vi "Master Control Loops.vi"() -> ()   [LabVIEW 2009]
uses:
  lib/Control Loop/Control Loop State.ctl
  lib/Data Access Objects/Control Loop/PID Controls.ctl
  lib/MixedMode/Mixed Mode States.ctl
  lib/MixedMode/Mixed Mode Convergence Status.ctl
  lib/MixedMode/Stiffness Matrix.ctl
  lib/Control Loop/Measurements.ctl
  lib/Data Access Objects/Metadata/LBCB Position.ctl
  lib/Control Loop/Limit Settings.ctl
  lib/Control Loop/Limit Matrix.ctl
  lib/Limits/Within Limits Matrix.ctl
  lib/Limits/Actuator Faults.ctl
  lib/Limits/Cart Disp Faults.ctl
  lib/Limits/Cart Force Faults.ctl
  lib/MixedMode/Target Data.ctl
  lib/MixedMode/Mixed Mode Cartesian Data.ctl
  lib/Autobalance/Autobalance Status Data.ctl
  lib/Apps/Yes No Button.ctl
  lib/Autobalance/Autobalance Stage.ctl
  lib/Autobalance/Autobalance Data Point.ctl
  lib/Data Access Objects/Mixed Mode/Force Control Parameters.ctl
  lib/Control Loop/Mixed Mode Hold Data type.ctl
  lib/Control Loop/Act & Cart Commands.ctl
  lib/Data Access Objects/Autobalance/Autobalance Control Parameters.ctl
  lib/Data Access Objects/Metadata/Cartesian Point.ctl
  lib/Global Data/Jacobian Stiffness Column.ctl
  lib/Global Data/Jacobian Stiffness Column Id.ctl
  lib/Control Loop/MM Result Actions.ctl
  lib/Data Access Objects/Metadata/DAO Actions.ctl
  lib/Apps/App Status Actions.ctl
  lib/Control Loop/Parameters Changes.ctl
  lib/Control Loop/Parameter Change States.ctl
  lib/Data Access Objects/Metadata/LBCB Number.ctl
  lib/MixedMode/Messages/Mixed Mode Command.ctl
  lib/MixedMode/Mixed Mode Command Action.ctl
  lib/MixedMode/Ramp Time Tuple.ctl
  lib/MixedMode/Messages/Mixed Mode Status.ctl
  lib/Autobalance/Autobalance State.ctl
  lib/Data Access Objects/Metadata/Persistant DAO Actions.ctl
  lib/Data Access Objects/Application/Number Of LBCBs.ctl
  lib/Global Data/Transactions/Dataset Transaction Id.ctl
  lib/Global Data/Transactions/Dataset Source.ctl
  lib/Global Data/Transactions/Dataset Type.ctl
  lib/Logging/Command or Stiffness Updates.ctl
  lib/Global Data/Command Or Stiffness Update Type.ctl
  lib/Data Access Objects/Global Cache/Global Cache.vi
  lib/Logging/LogFileType.ctl
  lib/DAQ IO/Daq Actions.ctl
  lib/Launcher/NoPanelAppTypes.ctl
  lib/Launcher/Launcher Actions.ctl
panel:
  out "MM Result Actions":T1
  out "Commands":T2[](array[typedef])
  out "Stiffness Jacobian Column":T3[](array[typedef])
  out "Target":T5[](array[typedef])
  out "Cart Individual Cmds":dbl[][](array[numeric])=[[0.015224103858920254, 0.016374115079328375, 0.0001743188568230551, 0.03971045114557009, 0.007082336209989981, 0.009859079687370698, 8.685887933911959, 1.9897804119684945, 4.857688782335148, 93.30834661628205, -5.911514458784602, -1.446477360303783]]
  out "Cart Meas. Disp & Forces":dbl[][](array[numeric])=[[0.015224103858920254, 0.016374115079328375, 0.0001743188568230551, 0.03971045114557009, 0.007082336209989981, 0.009859079687370698, 8.685887933911959, 1.9897804119684945, 4.857688782335148, 93.30834661628205, -5.911514458784602, -1.446477360303783]]
  out "Force Groups":T6[](array[typedef])
  in  "AB Parameters":T7={"Number of Samples"=0, "Delay After Cmd"=0, "Maximum Command"=0.0, "1/4 Linear Range"=0.5}
  out "Increment Limits":T2[](array[typedef])
  out "Hold Data":T8[](array[typedef])
  in  "L2 Ctrl Loop In Actuator":dbl[](array[numeric])
  out "Rigid Connection":bool
  out "Force Parameters":T9
  out "Stiffness Limits":dbl[][][](array[numeric])
  out "L2 Autobalance Out":T10[](array[typedef])
  out "L2 Cmd  Volts":dbl[](array[numeric])
  out "L2 Ctrl Loop Out Actuator":dbl[](array[numeric])=[0.012801822908652838, 0.012801822908652838, 7.98290599846041e-06, 8.154359441903125e-06, 8.154359441903125e-06, 8.154359441903125e-06]
  in  "Monitor Loop Time":u32
  in  "Volts LVDT & LC":dbl[][](array[numeric])
  out "L1 Autobalance Out":T10[](array[typedef])
  out "Collecting DAQ Samples":bool
  out "DAQ Volts":dbl[](array[numeric])=[-5.059315779335383, -5.016629198362524, -5.097891313865665, -5.092890991738198, -5.1138932889519, -4.974194835814303, 0.24442110332308561, 0.2508540081873783, -0.00045656932832031883, -0.0010919008583725697, -0.001119467422792373, -0.001138029771633142, 0.051584220664617125, 0.05637080163747566, -0.0007913138656640637, 0.023009008261802286, -0.021593288951899364, 0.0027051641856972383, -5.059665406563526, -5.018353952939143, -5.097893414204858, -5.0928919356893525, -5.11389113151188, -4.974191443340161, 0.24267296718237016, 0.2422302353042843, -0.0004670710242903981, -0.0011032282722249686, -0.0010935781425555466, -0.0010973200819313358, 0.05123459343647403, 0.05464604706085686, -0.0007934142048580796, 0.02300806431064792, -0.02159113151187963, 0.0027085566598390553, 0.048884220664617124, 0.04853459343647403, 0.050170801637475664, 0.04844604706085686, -9.131386566406377e-05, -9.341420485807962e-05]
  in  "Volt Logger Time":u32
  out "All Stopped":bool
  out "Previous Target":T14[](array[typedef])
  out "Iterative Target":T5[](array[typedef])
  out "Mixed Mode":i32
  out "Status Changes":i32
  out "L2 Control Rate":i32
  out "DAQ Started":bool
  out "Current Target":T5[](array[typedef])
  out "Logging Directory":path
  out "Auto Balance Error Tolerance":dbl[][](array[numeric])=[[0.01, 0.01, 0.01, 0.01, 0.01, 0.01]]
  in  "Hold Period":bool
  in  "Averaging":bool
  out "L1 Ctrl Loop State":T15
  out "Max Increment":dbl[][](array[numeric])
  out "Jacobian Gain":dbl[][](array[numeric])
  out "Force Error Range":dbl[][](array[numeric])
  out "L2 I Gain":dbl[](array[numeric])=[0.3, 0.3, 0.3, 0.3, 0.3, 0.3]
  in  "L2 PID On":bool
  in  "Limits Check":T16[](array[typedef])
  out "L2 P Gain":dbl[](array[numeric])
  out "L2 I Const":dbl[](array[numeric])
  in  "Ramp Time":u32
  out "Limits":T20[](array[typedef])
  out "Position":T22[](array[typedef])
  out "Measurements":T23[](array[typedef])
  out "Stiffness Jacobian":cluster{T24}[](array[cluster])
  out "Convergence Status":T25[](array[typedef])
  out "MixedModeStates":T26
  out "PID Control":T27[](array[typedef])
  in  "L1 PID On":bool
  out "L1 P Gain":dbl[](array[numeric])
  out "L1 I Gain":dbl[](array[numeric])=[0.3, 0.3, 0.3, 0.3, 0.3, 0.3]
  out "L1 I Const":dbl[](array[numeric])
  out "LBCB 1 Control Loop Force Limit":bool
  out "L2 Ctrl Loop State":T15
  out "L1 Cmd  Volts":dbl[](array[numeric])
  out "L1 Ctrl Loop Out Actuator":dbl[](array[numeric])=[0.012801822908652838, 0.012801822908652838, 7.98290599846041e-06, 8.154359441903125e-06, 8.154359441903125e-06, 8.154359441903125e-06]
  out "L1 Control Rate":i32=50 caption="Control Rate"
  in  "L1 Ctrl Loop In Actuator":dbl[](array[numeric])
  out "Number of \nExternal \nChannels":i32
  out "DAQ Enabled":bool
  in  "App Running":bool
  out "DAQ Rate":i32=2 caption="Control Rate"
  out "Servo Error":dbl[][](array[numeric])=[[-0.014471871278962644, -0.0027477897622864888, 0.03594582291831433, -0.006177356244415369, -0.000527948512754489, 0.04718526152757189]]
  out "Actuator Meas. Disp & Forces":dbl[][](array[numeric])=[[0.015224103858920254, 0.016374115079328375, 0.0001743188568230551, 0.03971045114557009, 0.007082336209989981, 0.009859079687370698, 8.685887933911959, 1.9897804119684945, 4.857688782335148, 93.30834661628205, -5.911514458784602, -1.446477360303783]]
  out "External Sensors":dbl[](array[numeric])
  out "DAQ Overflow":bool
  # "(Volts)"
  # "Cmd"
  # "Servo"
  # "Cmd"
  # "Servo"
  # "Cmd"
  # "Servo"
  # "Cmd"
  # "Servo"
  # "(inch)"
  # "X"
  # "(inch)"
  # "Y"
  # "(inch)"
  # "Z"
  # "Xglobal = T*Xlocal"
  # "Continuous"
  # "Hold"
types:
  T1 = typedef "MM Result Actions.ctl" = enum16{"Nop", "Set Command", "Check Limits", "Send Command", "Store Prev Reading", "Averaging On", "Averaging Off", "Hold On", "Hold Off", "PID Hold On", "PID Hold Off", "Clear Increment Faults", "Set Initial Position"}
  T2 = typedef "Act & Cart Commands.ctl" = cluster{"Act Cmd":dbl[], "Cart Cmd":dbl[]}
  T3 = typedef "Jacobian Stiffness Column.ctl" = cluster{"Id":T4, "Column":dbl[]}
  T4 = typedef "Jacobian Stiffness Column Id.ctl" = enum16{"dDx", "dDy", "dDz", "dRx", "dRy", "dRz"}
  T5 = typedef "Target Data.ctl" = cluster{"Displacements":dbl[], "Command Type":enum16{"<None>", "Displacement", "Force"}[], "Forces":dbl[]}
  T6 = typedef "Cartesian Point.ctl" = cluster{"Dx":dbl, "Dy":dbl, "Dz":dbl, "Rx":dbl, "Ry":dbl, "Rz":dbl}
  T7 = typedef "Autobalance Control Parameters.ctl" = cluster{"Number of Samples":i32, "Delay After Cmd":i32, "Maximum Command":dbl, "1/4 Linear Range":dbl}
  T8 = typedef "Mixed Mode Hold Data type.ctl" = cluster{"Displacements":dbl[], "Forces":dbl[], "Displacement \nCommands":dbl[]}
  T9 = typedef "Force Control Parameters.ctl" = cluster{"Use Force Error Range Ratios":bool, "Use Group Priorities":bool, "Multi Command Update":bool, "Steps per Stiffness \nMeasurement":i32}
  T10 = typedef "Autobalance Status Data.ctl" = cluster{"IsBalanced":T11, "Autobalance Stage":T12, "High":T13, "Low":T13, "Balanced \nCmd":dbl}
  T11 = typedef "Yes No Button.ctl" = bool
  T12 = typedef "Autobalance Stage.ctl" = enum16{"Coarse", "Fine", "Backing Up", "Done"}
  T13 = typedef "Autobalance Data Point.ctl" = cluster{"cCmd":dbl, "cServo":dbl, "pCmd":dbl, "pServo":dbl}
  T14 = typedef "Mixed Mode Cartesian Data.ctl" = cluster{"Displacements":dbl[], "Forces":dbl[]}
  T15 = typedef "Control Loop State.ctl" = enum16{"Idle", "Off", "Reset Autobalancing", "Autobalancing", "Set Command", "Ready for Control", "On"}
  T16 = typedef "Within Limits Matrix.ctl" = cluster{"Act Disp":T17, "Act Force":T17, "Act Incr":T17, "Cart Disp":T18, "Cart Force":T19, "Cart Incr":T18}
  T17 = typedef "Actuator Faults.ctl" = cluster{"X1":bool, "X2":bool, "Y1":bool, "Z1":bool, "Z2":bool, "Z3":bool}
  T18 = typedef "Cart Disp Faults.ctl" = cluster{"Dx":bool, "Dy":bool, "Dz":bool, "Rx":bool, "Ry":bool, "Rz":bool}
  T19 = typedef "Cart Force Faults.ctl" = cluster{"Fx":bool, "Fy":bool, "Fz":bool, "Mx":bool, "My":bool, "Mz":bool}
  T20 = typedef "Limit Settings.ctl" = cluster{"Actuator Force Limits":T21, "Actuator Stroke Limits":T21, "Cartesian Disp Limit":T21, "Cartesian Force Limit":T21, "Command Voltage Limit":T21}
  T21 = typedef "Limit Matrix.ctl" = dbl[][]
  T22 = typedef "LBCB Position.ctl" = cluster{"Motion Center":dbl[], "Transformation Matrix":dbl[][]}
  T23 = typedef "Measurements.ctl" = cluster{"Act Disp":dbl[], "Act Forces":dbl[], "Cart Disp":dbl[], "Cart Forces":dbl[]}
  T24 = typedef "Stiffness Matrix.ctl" = dbl[][]
  T25 = typedef "Mixed Mode Convergence Status.ctl" = cluster{"IsConverged":bool[], "Force Errors":dbl[], "Controlling DOF":bool[]}
  T26 = typedef "Mixed Mode States.ctl" = enum16{"Init", "Wait For DAQ", "Idle", "Start Initial Position", "Initial Position", "Start Initial Ramp", "Run Initial Ramp", "Start Iterative Stage", "Convergence Check", "Update Stiffness Jacobian", "Update Command", "Start Iterative Ramp", "Run Iterative Ramp", "Start Iterative Stabilize", "Iterative Stabilize", "Start Iterative Holding", "Iterative Holding", "Start Stabilize", "Stabilize", "Start Hold", "Holding", "Done", "Aborting", "Exit", "Nop"}
  T27 = typedef "PID Controls.ctl" = cluster{"I-Control":bool, "Ctrl Mode":bool}
  T28 = typedef "Command Or Stiffness Update Type.ctl" = cluster{"Target":T5[], "Stiffness":T3[], "Command || Stiffness Update":T29}
  T29 = typedef "Command or Stiffness Updates.ctl" = enum16{"Command Update", "Iterative Command Update", "Stiffness Update"}
  T30 = typedef "Dataset Transaction Id.ctl" = cluster{"Dataset Source":T31, "Dataset Type":T32, "Hold":T11, "Volts":T11, "Tag":string}
  T31 = typedef "Dataset Source.ctl" = enum16{"LBCB 1", "LBCB 2", "Combined", "External Sensors"}
  T32 = typedef "Dataset Type.ctl" = enum16{"LVDT", "Load Cell", "Actuator Command", "Servo Error", "Displacement Command", "Displacement", "Force"}
  T33 = typedef "Number Of LBCBs.ctl" = enum16{"1", "2"}
  T34 = cluster{"Act Disp":dbl[], "Act Forces":dbl[], "Cart Disp":dbl[], "Cart Forces":dbl[]}
  T35 = typedef "LBCB Number.ctl" = enum16{"LBCB1", "LBCB2"}
  T36 = typedef "Persistant DAO Actions.ctl" = enum16{"Init", "Get", "Set", "Load", "Save"}
  T37 = typedef "Autobalance State.ctl" = enum16{"Init", "Send High ", "Wait High", "Read High Start", "Read High", "Send Low", "Wait Low", "Read Low Start", "Read Low", "Publish", "Calculate", "Done"}
  T38 = typedef "Ramp Time Tuple.ctl" = cluster{"Ramp":dbl, "Stab":dbl, "Hold":dbl}
  T39 = typedef "Mixed Mode Command Action.ctl" = enum16{"Start Command", "Stop", "Exit", "No Op", "Start Acquisition", "Measure Initial Position"}
  T40 = typedef "Mixed Mode Status.ctl" = cluster{"LBCB Target":T5[], "MixedModeStates":T26, "LBCB Convergence":T25[], "LBCB Measurements":T14[]}
  T41 = typedef "Mixed Mode Command.ctl" = cluster{"Command":T39, "Ramp Times":cluster{"Initial":T38, "Iterative":T38}, "LBCB1":T5, "LBCB2":T5}
  T42 = typedef "Parameters Changes.ctl" = cluster{"Change State":T43, "LBCB Number":T35}
  T43 = typedef "Parameter Change States.ctl" = enum16{"Mixed Mode", "Control Loop", "Limits", "Application", "Stiffness Jacobian", "Start DAQ", "Reset Auto-Balance", "Set Command", "Enable Control", "Disable Control", "Position", "Stop Application"}
  T44 = typedef "DAO Actions.ctl" = enum16{"Init", "Get", "Set"}
  T45 = typedef "Actuator Matrix.ctl" = cluster{"Lower":T46, "Upper":T46}
  T46 = typedef "Actuator Point.ctl" = cluster{"X1":dbl, "X2":dbl, "Y1":dbl, "Z1":dbl, "Z2":dbl, "Z3":dbl}
  T47 = typedef "Cartesian Matrix.ctl" = cluster{"Lower":T6, "Upper":T6}
  T48 = typedef "App Parameters.ctl" = cluster{"Monitor Loop":T49, "Ramp Time":T49, "Log Loop":T49, "TCP to DAQ":T49, "Logging Directory":path, "Log File Size (MBytes)":i64, "Volt Logging Loop":T49, "2 LBCB Archiving Mode":bool}
  T49 = typedef "Timing Parameters.ctl" = cluster{"Interval":dbl, "Rate ":dbl}
  T50 = typedef "LBCB Settings.ctl" = cluster{"Size":T51, "Type":T52}
  T51 = typedef "LBCB Size.ctl" = enum16{"1/5th-scale LBCB", "Full-scale LBCB", "Portable LBCB"}
  T52 = typedef "LBCB Type.ctl" = enum16{"X Actuators On The Left", "X Actuators On The Right"}
  T53 = typedef "Cartesian Force Vector.ctl" = cluster{"Fx":dbl, "Fy":dbl, "Fz":dbl, "Mx":dbl, "My":dbl, "Mz":dbl}
  T54 = typedef "Calibration Settings.ctl" = cluster{"Command Sensitivity":dbl[], "Servo Error Offset":dbl[], "LVDT Sensitivity":dbl[], "LVDT Offset":dbl[], "Load Cell Offsets":dbl[], "Load Cell Sensitivity":dbl[]}
  T55 = typedef "App Status Actions.ctl" = enum16{"Init", "Get Status", "Running", "Control", "Autobalanced", "Data Acquisition", "Set App State", "DAQ Started", "Set LBCB State", "Set All", "Set Cont Logging", "Set Step Logging", "Set MM Logging", "Set Volt Logging", "Set DAQ Link"}
  T56 = typedef "Ramp Time Input.ctl" = cluster{"Directional":T57, "Iterative":T57}
  T57 = typedef "Ramp Control.ctl" = cluster{"Ramp":dbl, "Stabilize":dbl, "Hold":dbl}
  T58 = typedef "App Status.ctl" = cluster{"Running":bool, "Controlling L2":bool, "Autobalance L2":bool, "Data Acquisition":bool, " App State":T59, "DAQ Started":bool, "LBCB 1 State":T60, "LBCB 2 State":T60, "Controlling L1":bool, "Autobalance L1":bool, "Continuous Logging":bool, "Step Logging":bool, "Voltage Logging":bool, "Mixed Mode Logging":bool, "DAQ Link":bool}
  T59 = typedef "AppStates.ctl" = enum16{"Starting OM", "Initializing Displays", "Setting up Archiving", "Setting Up DAQ Channels", "Start DAQ", "DAQ Starting", "Controlling LBCBs", "Stopping OM"}
  T60 = typedef "Lbcb Control Loop States.ctl" = enum16{"Idle", "Start Selected", "Load Last Command", "Start Autobalancing", "Autobalancing", "Control Loop Initialized", "Control Enabled"}
  T61 = cluster{"Act Disp":dbl[], "Act Forces":dbl[], "Cart Disp":dbl[], "Cart Forces":dbl[]}[]
  T62 = typedef "Daq Actions.ctl" = enum16{"Init", "Send Commands", "Get Responses", "Stop"}
  T63 = enum16{"open", "replace", "create", "open or create", "replace or create", "replace or create with confirmation"}
  T64 = typedef "LogFileType.ctl" = enum16{"Continuous", "Step", "Volts", "Offsets", "DLL  Errors", "Snapshot", "Commands", "StiffnessUpdates", "End List"}
  T65 = typedef "NoPanelAppTypes.ctl" = enum16{"NTCP Socket", "Data Archiving", "DAQ Link", "Control Loops", "Cmd Disp Diffs", "LBCB Data", "Limits", "Mixed Mode Widget", "Offsets"}
  T66 = typedef "Launcher Actions.ctl" = enum16{"Launch", "Stop All", "Stop", "Kill", "Running?", "Init"}
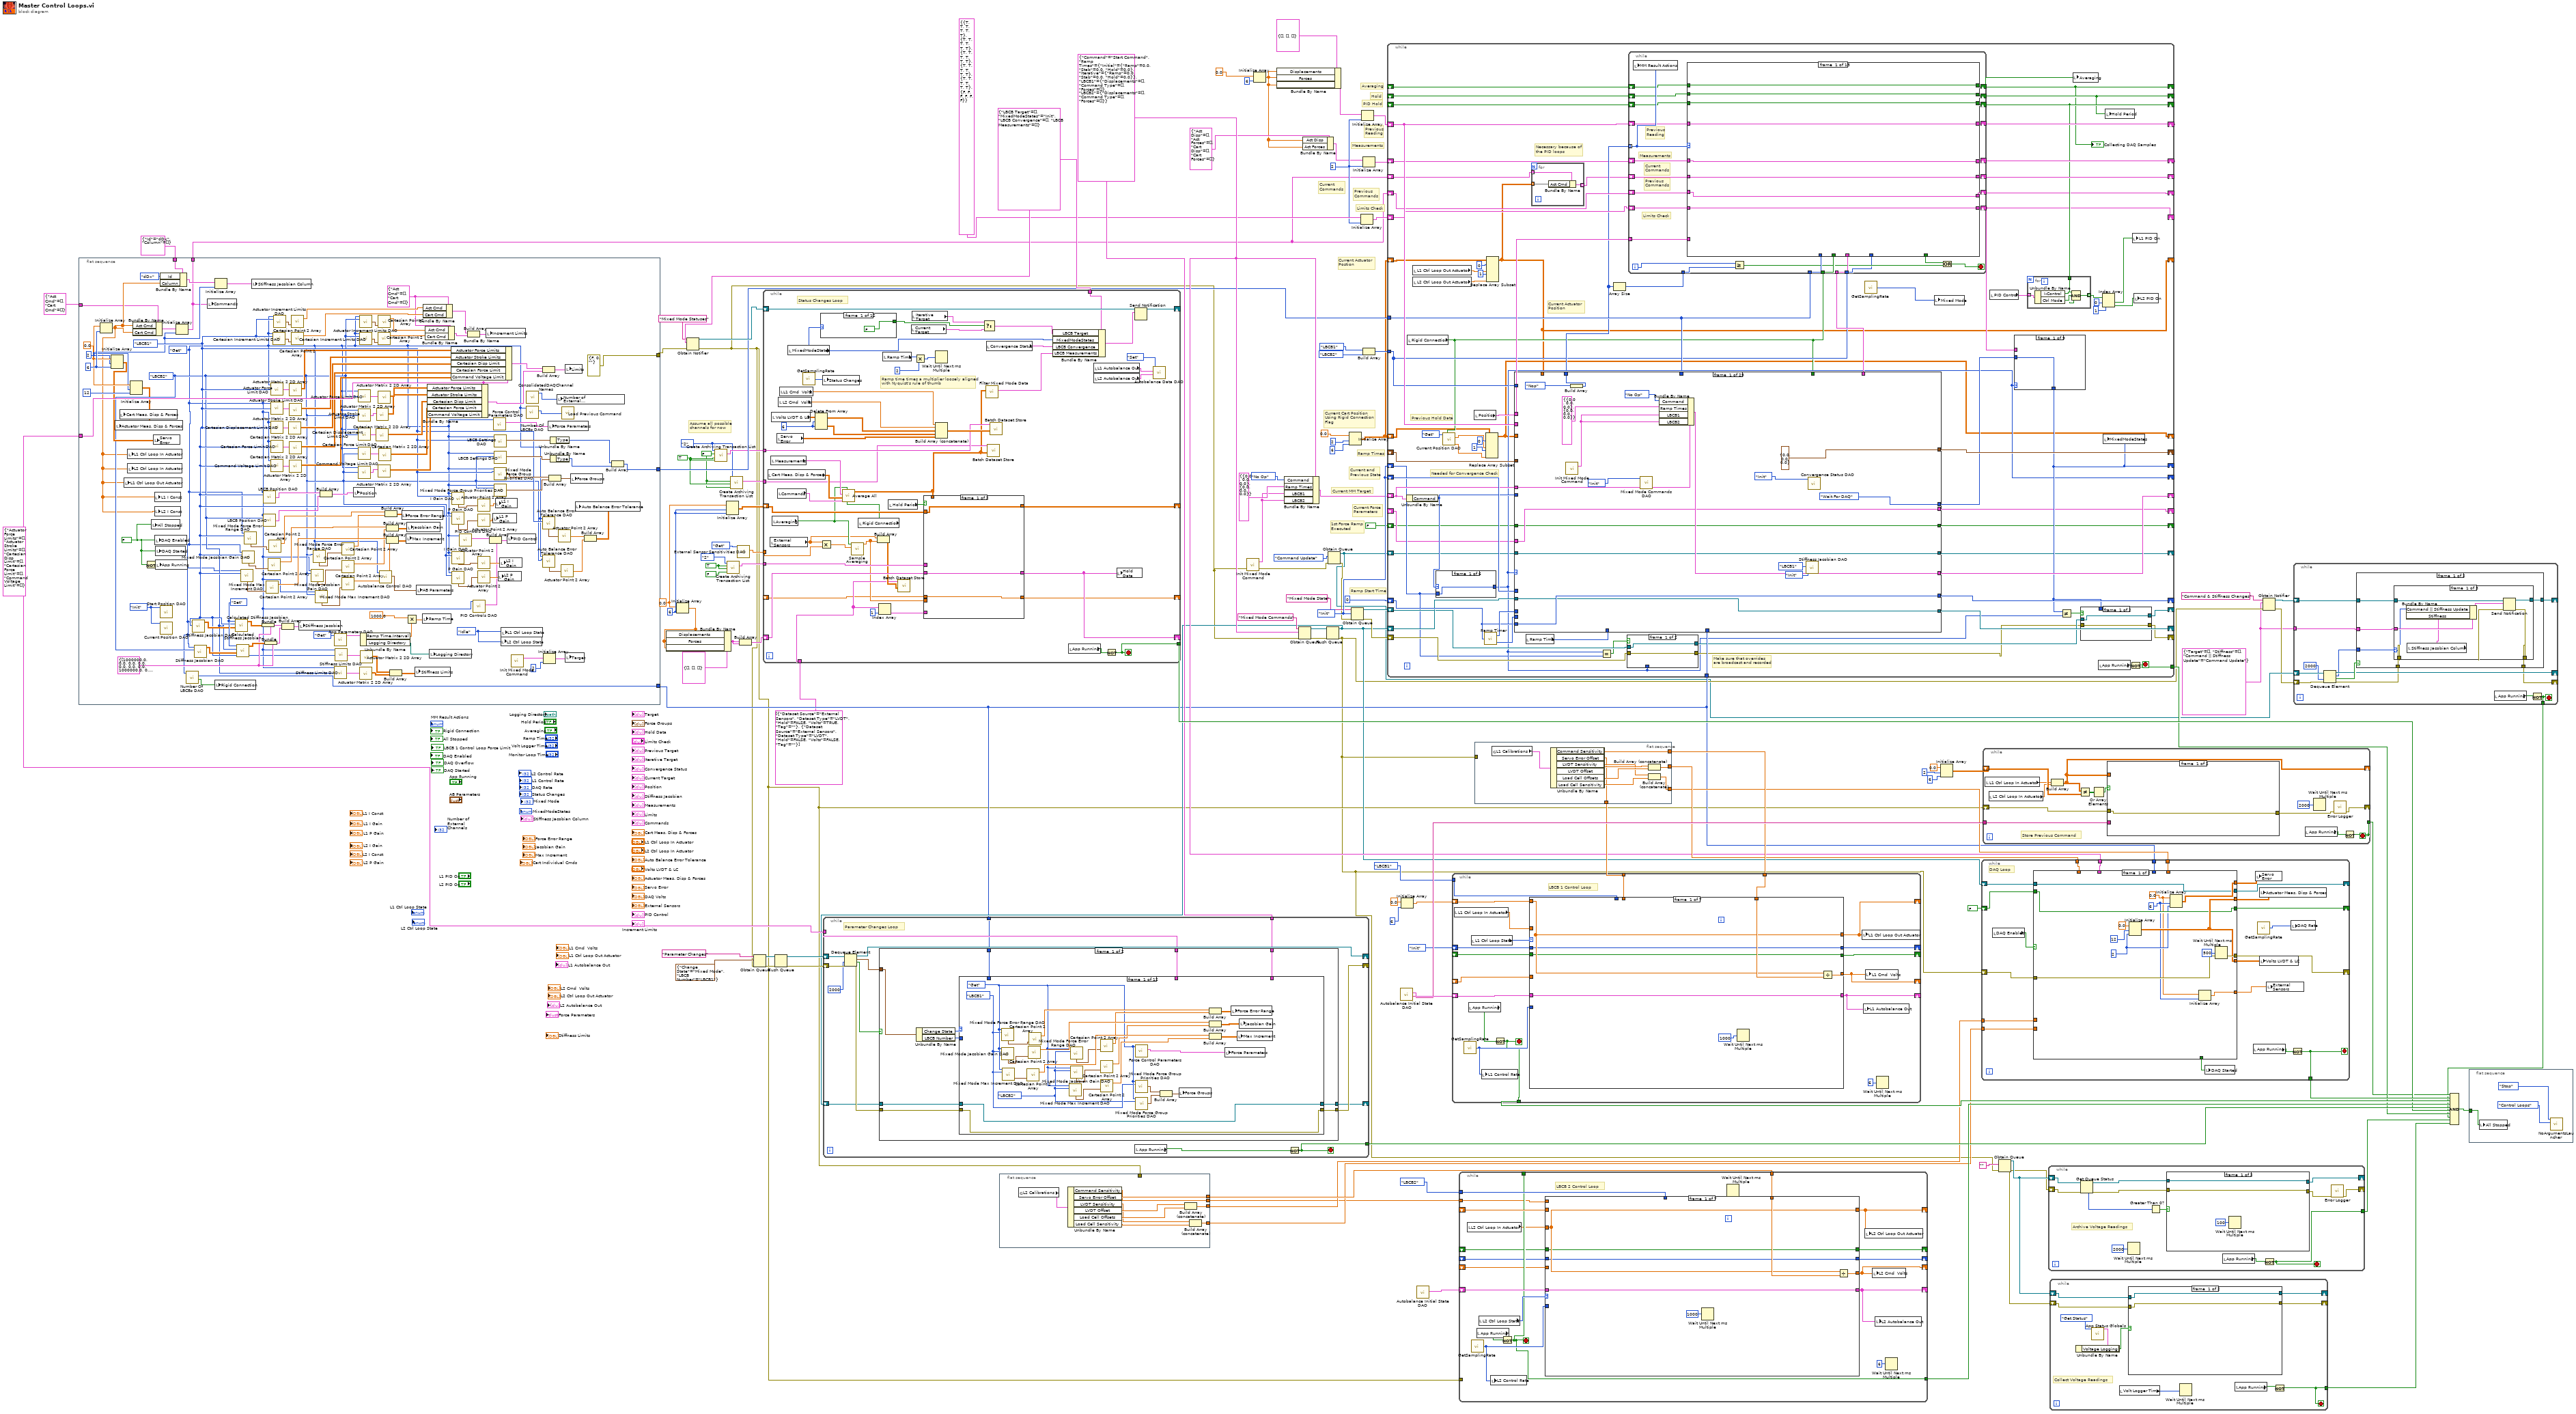
[diagram p0: block diagram]
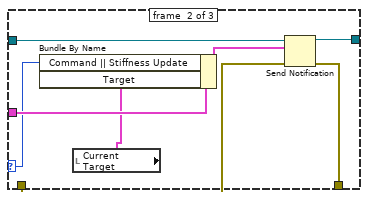
[diagram p2: hidden frame]
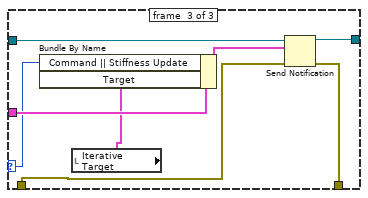
[diagram p3: hidden frame]
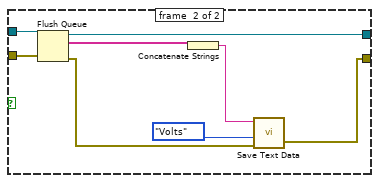
[diagram p5: hidden frame]
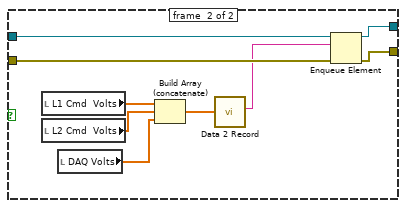
[diagram p6: hidden frame]
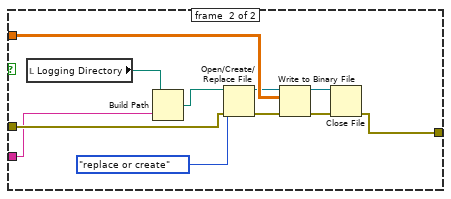
[diagram p7: hidden frame]
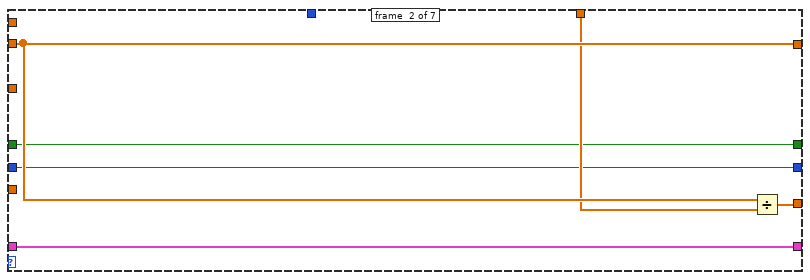
[diagram p8: hidden frame]
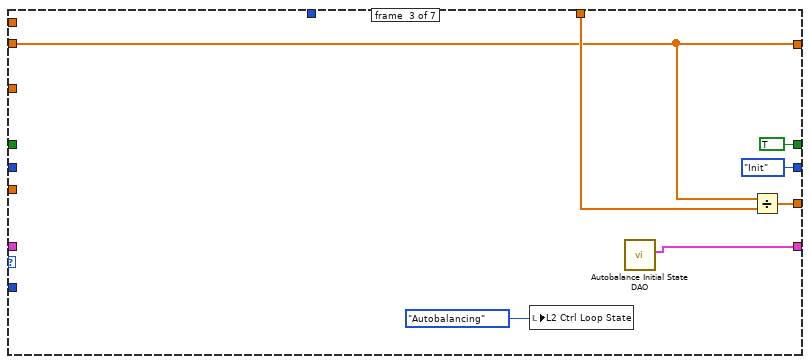
[diagram p9: hidden frame]
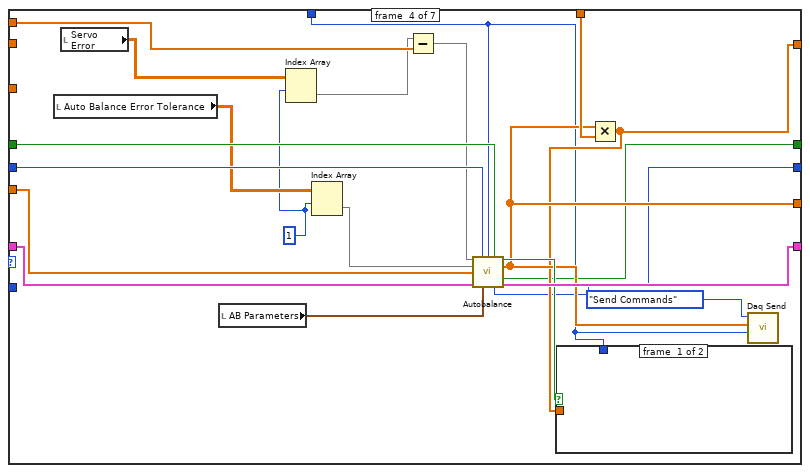
[diagram p10: hidden frame]
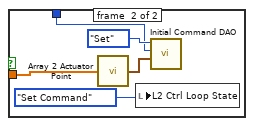
[diagram p11: hidden frame]
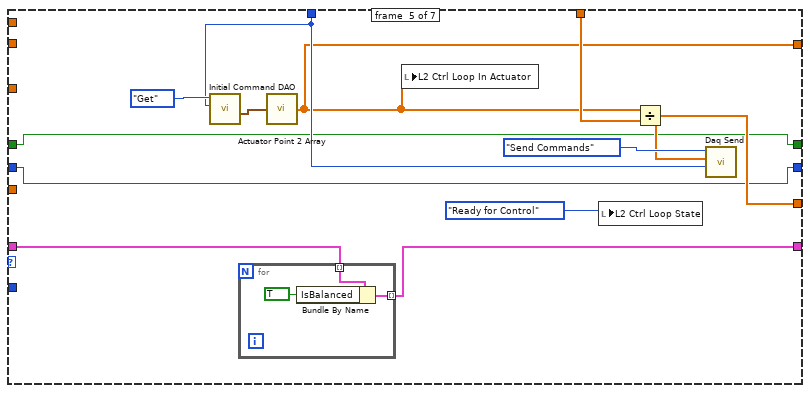
[diagram p12: hidden frame]
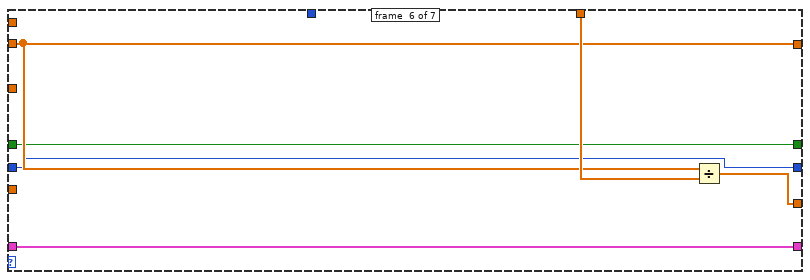
[diagram p13: hidden frame]
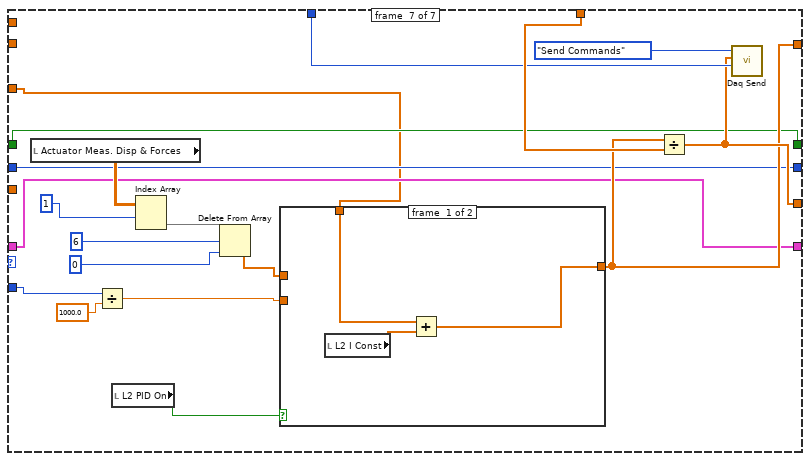
[diagram p14: hidden frame]
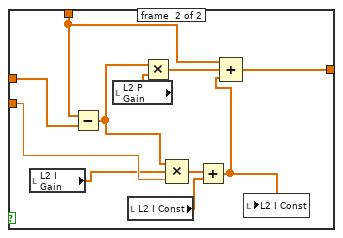
[diagram p15: hidden frame]
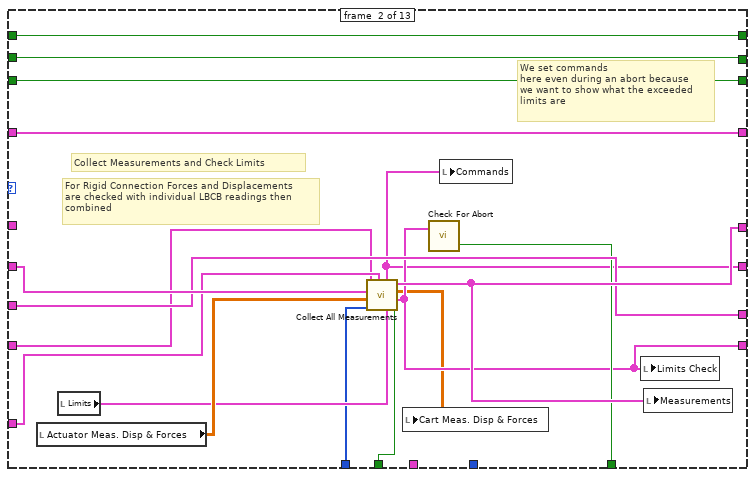
[diagram p16: hidden frame]
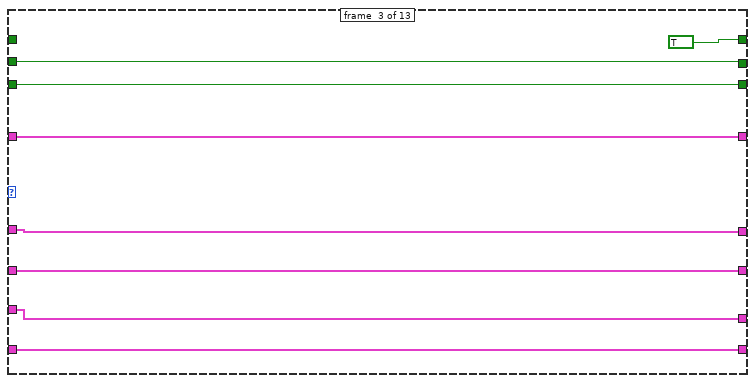
[diagram p17: hidden frame]
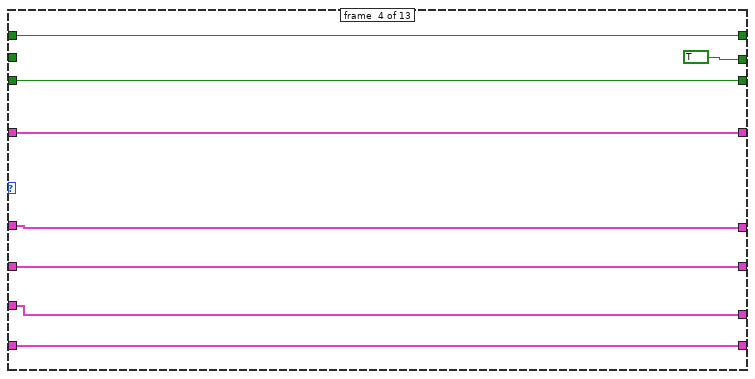
[diagram p18: hidden frame]
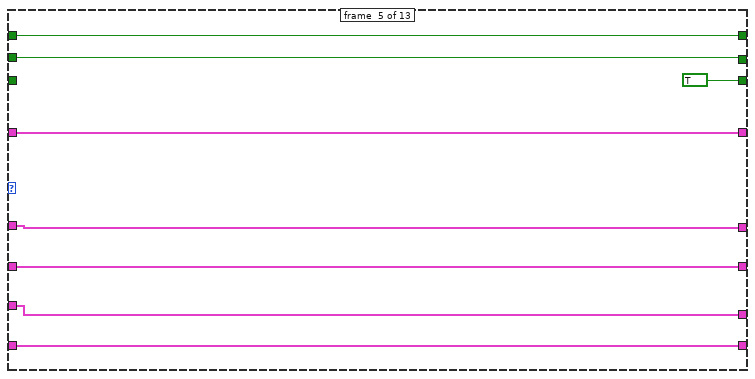
[diagram p19: hidden frame]
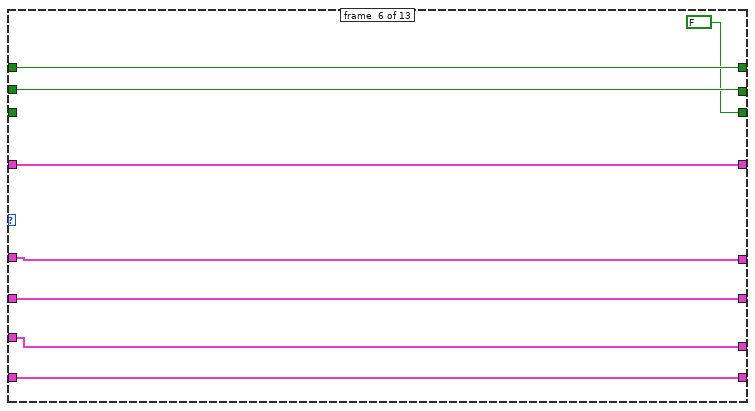
[diagram p20: hidden frame]
diagram:
  w3 = T28 {"Target"=[], "Stiffness"=[], "Command || Stiffness Update"=enum."Command Update"} ("Command || Stiffness Update")
  w20 = TRUE ("Combined LBCBs")
  w17 = Number_Of_LBCBs."2" ("Number of LBCBs")
  w13 = T11 TRUE ("Hold")
  w18 = T11 FALSE ("Hold")
  w23 = 0.0 ("element")
  w24 = 6 ("dimension size")
  w44 = 2 ("dimension size")
  w66 = T20 {"Actuator Force Limits"=[], "Actuator Stroke Limits"=[], "Cartesian Disp Limit"=[], "Cartesian Force Limit"=[], "Command Voltage Limit"=[]} ("L1  Limits")
  w104 = T40 {"LBCB Target"=[], "MixedModeStates"=enum."Init", "LBCB Convergence"=[], "LBCB Measurements"=[]} ("Mixed Mode Status")
  w64 = T41 {"Command"=enum."Start Command", "Ramp Times"={"Initial"={"Ramp"=0.0, "Stab"=0.0, "Hold"=0.0}, "Iterative"={"Ramp"=0.0, "Stab"=0.0, "Hold"=0.0}}, "LBCB1"={"Displacements"=[], "Command Type"=[], "Forces"=[]}, "LBCB2"={"Displacements"=[], "Command Type"=[], "Forces"=[]}} ("Mixed Mode Command")
  w111 = Mixed_Mode_States."Init" ("MixedModeStates")
  # "Assume all possible\nchannels for now"
  # "Current Actuator\nPostion"
  # "Current Cart Position\nUsing Rigid Connection\nFlag"
  # "1st Force Ramp\nExecuted"
  # "Current Force\nParameters"
  # "Previous\nCommands"
  # "Limits Check"
  # "Ramp Start Time"
  # "PID Hold"
  # "Hold"
  # "Averaging"
  # "Previous\nReading"
  # "Current \nCommands"
  # "Measurements"
  # "Current MM Target"
  # "Current and\nPrevious State"
  # "Ramp Times"
  n1 = flat-sequence {
    tunnel: [errorcluster {"status"=FALSE, "code"=0, "source"=""} ("error out")] -> w69
    tunnel: w66 -> [w207]
    tunnel: [w156] -> w46
    tunnel: [w151] -> w45
    tunnel: [w116] -> w43
    tunnel: T3 {"Id"=enum."dDx", "Column"=[]} ("Jacobian Stiffness Column") -> [w125]
    tunnel: T2 {"Act Cmd"=[], "Cart Cmd"=[]} ("Data") -> [w120]
    frame #0 {
      w127 = DAO_Actions."Init" ("DAO Actions")
      w129 = T2 {"Act Cmd"=[], "Cart Cmd"=[]} ("Data")
      w173 = cluster{T24} {[[1000000.0, 0.0, 0.0, 0.0, 0.0, 0.0], [0.0, 1000000.0, 0.0, 0.0, 0.0, 0.0], [0.0, 0.0, 1000000.0, 0.0, 0.0, 0.0], [0.0, 0.0, 0.0, 1000000.0, 0.0, 0.0], [0.0, 0.0, 0.0, 0.0, 1000000.0, 0.0], [0.0, 0.0, 0.0, 0.0, 0.0, 1000000.0]]} ("Cluster")
      w126 = 2 ("dimension size")
      w210 = Control_Loop_State."Idle" ("L1 Ctrl Loop State")
      w177 = 6 ("dimension size")
      w176 = 0.0 ("element")
      w137 = LBCB_Number."LBCB2" ("ID")
      w138 = LBCB_Number."LBCB1" ("ID")
      w136 = Persistant_DAO_Actions."Get" ("Actuator Force Limit Actions")
      w214 = FALSE
      w230 = Persistant_DAO_Actions."Set" ("Actions")
      n2 = Initialize Array(w176, w177) -> (w123:dbl[])
      n3 = Initialize Array(w176, w126, w177) -> (w141:dbl[][])
      n4 = local write "L1 Ctrl Loop Out Actuator"(w123) -> ()
      n5 = local write "L1 Ctrl Loop In Actuator"(w123) -> ()
      n6 = local write "L2 Ctrl Loop In Actuator"(w123) -> ()
      n7 = Initialize Array(w176, w126, 12 ("dimension size")) -> (w128:dbl[][])
      n8 = local write "Actuator Meas. Disp & Forces"(w128) -> ()
      n9 = local write "Cart Meas. Disp & Forces"(w128) -> ()
      n10 = Bundle By Name(cluster=w120, "Act Cmd"=w123, "Cart Cmd"=w123) -> (w150:T2)
      n11 = Not(x=w214) -> (.not. x?=w228:bool)
      n12 = local write "All Stopped"(w214) -> ()
      n13 = local write "Servo Error"(w141) -> ()
      n14 = local write "L1 I Const"(w123) -> ()
      n15 = local write "L2 I Const"(w123) -> ()
      n16 = local write "DAQ Enabled"(w214) -> ()
      n17 = local write "DAQ Started"(w214) -> ()
      n18 = local write "App Running"(w228) -> ()
      n19 = call "Start Position DAO.vi"("DAO Actions"=w127) -> ()  [unwired: 9 in, 2 out]
      n20 = call "Current Position DAO.vi"("Actions"=w127) -> ()  [unwired: 9 in, 2 out]
      n21 = Bundle By Name(cluster=w125, "Id"=Jacobian_Stiffness_Column_Id."dDx", "Column"=w123) -> (w122:T3)
      n22 = Initialize Array(w150, w126) -> (w116:T2[])
      n23 = call "Number Of LBCBs DAO.vi"("Actions"=w136) -> ("Rigid Connection Out"=w157:bool, "Number of\nLBCBs Out"=w156:T33)  [unwired: 4 in, 5 out]
      n24 = call "Stiffness Jacobian DAO.vi"("LBCB Number"=w138, "Actions"=w136) -> ("Stiffness Jacobian Out"=w229:T24)  [unwired: 3 in, 6 out]
      n25 = call "Stiffness Jacobian DAO.vi"("LBCB Number"=w137, "Actions"=w136) -> ("Stiffness Jacobian Out"=w231:T24)  [unwired: 3 in, 6 out]
      n26 = local write "Commands"(w116) -> ()
      n27 = local write "Rigid Connection"(w157) -> ()
      n28 = Initialize Array(w122, w126) -> (w121:T3[])
      n29 = call "Calculated Stiffness Jacobian.vi"("Stiffness Jacobian In"=w229, "LBCB Number"=w138, "Actions"=w230) -> ("Stiffness Jacobian Out"=w175:T24)  [unwired: 1 in, 7 out]
      n30 = call "Calculated Stiffness Jacobian.vi"("Stiffness Jacobian In"=w231, "LBCB Number"=w137, "Actions"=w230) -> ("Stiffness Jacobian Out"=w174:T24)  [unwired: 1 in, 7 out]
      n31 = call "Mixed Mode Max Increment DAO.vi"("Max Increment Actions"=w136, "LBCB Number"=w138) -> ("Max Increment Out"=w238:T6)  [unwired: 3 in, 10 out]
      n32 = call "Mixed Mode Jacobian Gain DAO.vi"("Jacobian Gain Actions"=w136, "LBCB Number"=w138) -> ("Jacobian Gain Out"=w237:T6)  [unwired: 3 in, 10 out]
      n33 = call "Mixed Mode Force Error Range DAO.vi"("Force Error Range Actions"=w136, "LBCB Number"=w138) -> ("Force Error Range Out"=w236:T6)  [unwired: 3 in, 10 out]
      n34 = local write "Stiffness Jacobian Column"(w121) -> ()
      n35 = Bundle(cluster=w173, w175) -> (w172:cluster{T24})
      n36 = call "LBCB Position DAO.vi"("LBCB Settings Actions"=w136, "LBCB Number"=w138) -> ("LBCB Position Output"=w235:T22)  [unwired: 3 in, 10 out]
      n37 = call "LBCB Position DAO.vi"("LBCB Settings Actions"=w136, "LBCB Number"=w137) -> ("LBCB Position Output"=w185:T22)  [unwired: 3 in, 10 out]
      n38 = Bundle(cluster=w173, w174) -> (w171:cluster{T24})
      n39 = call "Cartesian Point 2 Array.vi"("Cart Disp"=w238) -> ("Array"=w232:dbl[])  [unwired: 2 out]
      n40 = call "Cartesian Point 2 Array.vi"("Cart Disp"=w237) -> ("Array"=w233:dbl[])  [unwired: 2 out]
      n41 = call "Cartesian Point 2 Array.vi"("Cart Disp"=w236) -> ("Array"=w234:dbl[])  [unwired: 2 out]
      n42 = call "Actuator Force Limit DAO.vi"("Actuator Force Limit Actions"=w136, "ID"=w138) -> ("Actuator Force Limits Out"=w206:T45)  [unwired: 3 in, 10 out]
      n43 = call "Actuator Stroke Limit DAO.vi"("Actuator Stroke Limit Actions"=w136, "ID"=w138) -> ("Actuator Stroke Limits Out"=w205:T45)  [unwired: 3 in, 10 out]
      n44 = call "Cartesian Displacement Limit DAO.vi"("Cartesian Displacement Limit Actions"=w136, "ID"=w138) -> ("Cartesian Displacement Out"=w200:T47)  [unwired: 3 in, 10 out]
      n45 = call "Cartesian Force Limit DAO.vi"("Cartesian Force Limit Actions"=w136, "ID"=w138) -> ("Cartesian Force Limit Out"=w199:T47)  [unwired: 3 in, 10 out]
      n46 = call "Command Voltage Limit DAO.vi"("Actuator Stroke Limit Actions"=w136, "ID"=w138) -> ("Command Voltage Limit Out"=w204:T45)  [unwired: 3 in, 10 out]
      n47 = call "Cartesian Increment Limits DAO.vi"("Actions"=w136, "LBCB Number"=w138) -> ("Inc Limits Out"=w149:T6)  [unwired: 11 in, 2 out]
      n48 = call "Actuator Increment Limits DAO.vi"("Actions"=w136, "LBCB Number"=w138) -> ("Inc Limits Out"=w140:T46)  [unwired: 11 in, 2 out]
      n49 = Build Array(w172, w171) -> (w170:cluster{T24}[])
      n50 = call "Cartesian Matrix 2 2D Array.vi"("Matrix In"=w200) -> ("Matrix Out"=w188:T21)  [unwired: 10 out]
      n51 = call "Actuator Matrix 2 2D Array.vi"("Matrix In"=w206) -> ("Matrix Out"=w203:T21)  [unwired: 10 out]
      n52 = call "Actuator Matrix 2 2D Array.vi"("Matrix In"=w205) -> ("Matrix Out"=w202:T21)  [unwired: 10 out]
      n53 = call "Cartesian Matrix 2 2D Array.vi"("Matrix In"=w199) -> ("Matrix Out"=w187:T21)  [unwired: 10 out]
      n54 = call "Actuator Matrix 2 2D Array.vi"("Matrix In"=w204) -> ("Matrix Out"=w201:T21)  [unwired: 10 out]
      n55 = call "Cartesian Point 2 Array.vi"("Cart Disp"=w149) -> ("Array"=w133:dbl[])  [unwired: 2 in]
      n56 = call "Cartesian Point 2 Array.vi"("Cart Disp"=w140) -> ("Array"=w135:dbl[])  [unwired: 2 in]
      n57 = local write "Stiffness Jacobian"(w170) -> ()
      n58 = call "Mixed Mode Jacobian Gain DAO.vi"("Jacobian Gain Actions"=w136, "LBCB Number"=w137) -> ("Jacobian Gain Out"=w212:T6)  [unwired: 3 in, 10 out]
      n59 = call "Mixed Mode Force Error Range DAO.vi"("Force Error Range Actions"=w136, "LBCB Number"=w137) -> ("Force Error Range Out"=w211:T6)  [unwired: 3 in, 10 out]
      n60 = call "Mixed Mode Max Increment DAO.vi"("Max Increment Actions"=w136, "LBCB Number"=w137) -> ("Max Increment Out"=w213:T6)  [unwired: 3 in, 10 out]
      n61 = Build Array(w235, w185) -> (w186:T22[])
      n62 = call "App Parameters DAO.vi"("Actions"=Persistant_DAO_Actions."Get") -> ("Application Timing and Logging Out"=w242:T48)  [unwired: 3 in, 7 out]
      n63 = call "Stiffness Limits DAO.vi"("Cartesian Force Limit Actions"=w136, "ID"=w137) -> ("Stiffness Limit Out"=w160:T47)  [unwired: 11 in, 2 out]
      n64 = call "Stiffness Limits DAO.vi"("Cartesian Force Limit Actions"=w136, "ID"=w138) -> ("Stiffness Limit Out"=w162:T47)  [unwired: 11 in, 2 out]
      n65 = call "Cartesian Point 2 Array.vi"("Cart Disp"=w211) -> ("Array"=w183:dbl[])  [unwired: 1 in, 1 out]
      n66 = call "Cartesian Point 2 Array.vi"("Cart Disp"=w212) -> ("Array"=w181:dbl[])  [unwired: 1 in, 1 out]
      n67 = call "Cartesian Point 2 Array.vi"("Cart Disp"=w213) -> ("Array"=w179:dbl[])  [unwired: 1 in, 1 out]
      n68 = local write "Position"(w186) -> ()
      n69 = call "Actuator Force Limit DAO.vi"("Actuator Force Limit Actions"=w136, "ID"=w137) -> ("Actuator Force Limits Out"=w198:T45)  [unwired: 3 in, 10 out]
      n70 = call "Actuator Stroke Limit DAO.vi"("Actuator Stroke Limit Actions"=w136, "ID"=w137) -> ("Actuator Stroke Limits Out"=w197:T45)  [unwired: 3 in, 10 out]
      n71 = call "Cartesian Displacement Limit DAO.vi"("Cartesian Displacement Limit Actions"=w136, "ID"=w137) -> ("Cartesian Displacement Out"=w196:T47)  [unwired: 3 in, 10 out]
      n72 = call "Cartesian Force Limit DAO.vi"("Cartesian Force Limit Actions"=w136, "ID"=w137) -> ("Cartesian Force Limit Out"=w195:T47)  [unwired: 3 in, 10 out]
      n73 = call "Command Voltage Limit DAO.vi"("Actuator Stroke Limit Actions"=w136, "ID"=w137) -> ("Command Voltage Limit Out"=w194:T45)  [unwired: 3 in, 10 out]
      n74 = call "Cartesian Increment Limits DAO.vi"("Actions"=w136, "LBCB Number"=w137) -> ("Inc Limits Out"=w148:T6)  [unwired: 11 in, 2 out]
      n75 = call "Actuator Increment Limits DAO.vi"("Actions"=w136, "LBCB Number"=w137) -> ("Inc Limits Out"=w139:T46)  [unwired: 11 in, 2 out]
      n76 = call "Actuator Matrix 2 2D Array.vi"("Matrix In"=w160) -> ("Matrix Out"=w159:T21)  [unwired: 10 out]
      n77 = Unbundle By Name(w242) -> ("Ramp Time.Interval"=w243:dbl, "Logging Directory"=w239:path)
      n78 = call "Actuator Matrix 2 2D Array.vi"("Matrix In"=w162) -> ("Matrix Out"=w161:T21)  [unwired: 10 out]
      n79 = call "Cartesian Matrix 2 2D Array.vi"("Matrix In"=w196) -> ("Matrix Out"=w191:T21)  [unwired: 10 out]
      n80 = call "Actuator Matrix 2 2D Array.vi"("Matrix In"=w197) -> ("Matrix Out"=w192:T21)  [unwired: 10 out]
      n81 = call "Cartesian Point 2 Array.vi"("Cart Disp"=w148) -> ("Array"=w132:dbl[])  [unwired: 2 in]
      n82 = call "Cartesian Point 2 Array.vi"("Cart Disp"=w139) -> ("Array"=w134:dbl[])  [unwired: 2 in]
      n83 = call "Actuator Matrix 2 2D Array.vi"("Matrix In"=w198) -> ("Matrix Out"=w193:T21)  [unwired: 10 out]
      n84 = call "Actuator Matrix 2 2D Array.vi"("Matrix In"=w194) -> ("Matrix Out"=w189:T21)  [unwired: 10 out]
      n85 = call "Cartesian Matrix 2 2D Array.vi"("Matrix In"=w195) -> ("Matrix Out"=w190:T21)  [unwired: 10 out]
      n86 = call "Autobalance Control DAO.vi"("Persistent DAO Actions"=w136) -> ("Autobalance Control Out"=w146:T7)  [unwired: 8 in, 2 out]
      n87 = Build Array(w234, w183) -> (w184:dbl[][])
      n88 = Build Array(w233, w181) -> (w182:dbl[][])
      n89 = Build Array(w232, w179) -> (w180:dbl[][])
      n90 = Build Array(w161, w159) -> (w158:dbl[][][])
      n91 = local write "Force Error Range"(w184) -> ()
      n92 = local write "Max Increment"(w180) -> ()
      n93 = Multiply(x=1000.0, y=w243) -> (x*y=w240:dbl)
      n94 = local write "Jacobian Gain"(w182) -> ()
      n95 = local write "Stiffness Limits"(w158) -> ()
      n96 = local write "AB Parameters"(w146) -> ()
      n97 = local write "Ramp Time"(w240) -> ()
      n98 = Bundle By Name(cluster=w129, "Act Cmd"=w135, "Cart Cmd"=w133) -> (w131:T2)
      n99 = Bundle By Name(cluster=w129, "Act Cmd"=w134, "Cart Cmd"=w132) -> (w130:T2)
      n100 = Bundle By Name(cluster=w207, "Actuator Force Limits"=w193, "Actuator Stroke Limits"=w192, "Cartesian Disp Limit"=w191, "Cartesian Force Limit"=w190, "Command Voltage Limit"=w189) -> (w166:T20)
      n101 = local write "Logging Directory"(w239) -> ()
      n102 = Bundle By Name(cluster=w207, "Actuator Force Limits"=w203, "Actuator Stroke Limits"=w202, "Cartesian Disp Limit"=w188, "Cartesian Force Limit"=w187, "Command Voltage Limit"=w201) -> (w208:T20)
      n103 = call "I Gain DAO.vi"("I Gain Actions"=w136, "LBCB Number"=w138) -> ("I Gain"=w224:T46)  [unwired: 3 in, 10 out]
      n104 = call "P Gain DAO.vi"("P Gain Actions"=w136, "LBCB Number"=w138) -> ("P Gain"=w225:T46)  [unwired: 3 in, 10 out]
      n105 = call "I Gain DAO.vi"("I Gain Actions"=w136, "LBCB Number"=w137) -> ("I Gain"=w227:T46)  [unwired: 3 in, 10 out]
      n106 = call "P Gain DAO.vi"("P Gain Actions"=w136, "LBCB Number"=w137) -> ("P Gain"=w226:T46)  [unwired: 3 in, 10 out]
      n107 = call "PID Controls DAO.vi"("Actions"=w136) -> ("PID Control  Out"=w165:T27)  [unwired: 3 in, 7 out]
      n108 = Build Array(w131, w130) -> (w147:T2[])
      n109 = call "PID Controls DAO.vi"("Actions"=w136) -> ("PID Control  Out"=w163:T27)  [unwired: 3 in, 7 out]
      n110 = call "Actuator Point 2 Array.vi"("Actuator Point"=w224) -> ("Array"=w223:dbl[])
      n111 = call "Actuator Point 2 Array.vi"("Actuator Point"=w225) -> ("Array"=w222:dbl[])
      n112 = call "Actuator Point 2 Array.vi"("Actuator Point"=w227) -> ("Array"=w221:dbl[])
      n113 = call "Actuator Point 2 Array.vi"("Actuator Point"=w226) -> ("Array"=w220:dbl[])
      n114 = local write "Increment Limits"(w147) -> ()
      n115 = Build Array(w165, w163) -> (w164:T27[])
      n116 = local write "L1 P Gain"(w222) -> ()
      n117 = call "Force Control Parameters DAO.vi"("DAO Actions"=w136) -> ("Force Control Parameters Out"=w142:T9)  [unwired: 8 in, 2 out]
      n118 = call "LBCB Settings DAO.vi"("LBCB Number"=w138, "Actions"=w136) -> ("LBCB Setting Out"=w154:T50)  [unwired: 3 in, 6 out]
      n119 = call "LBCB Settings DAO.vi"("LBCB Number"=w137, "Actions"=w136) -> ("LBCB Setting Out"=w155:T50)  [unwired: 3 in, 6 out]
      n120 = call "Mixed Mode Force Group Priorities DAO.vi"("Force Error Range Actions"=w136, "LBCB Number"=w138) -> ("Force Group Priorities Out"=w145:T53)  [unwired: 11 in, 2 out]
      n121 = call "Mixed Mode Force Group Priorities DAO.vi"("Force Error Range Actions"=w136, "LBCB Number"=w137) -> ("Force Group Priorities Out"=w144:T53)  [unwired: 11 in, 2 out]
      n122 = local write "L1 I Gain"(w223) -> ()
      n123 = local write "L2 P Gain"(w220) -> ()
      n124 = local write "L2 I Gain"(w221) -> ()
      n125 = local write "L2 Ctrl Loop State"(w210) -> ()
      n126 = local write "L1 Ctrl Loop State"(w210) -> ()
      n127 = local write "PID Control"(w164) -> ()
      n128 = call "Init Mixed Mode Command.vi"() -> ("Command Data"=w119:T5)  [unwired: 2 in, 1 out]
      n129 = call "Number Of LBCBs DAO.vi"("Actions"=w136) -> ("Number of\nLBCBs Out"=w209:T33)  [unwired: 4 in, 6 out]
      n130 = call "ConsolidatedDAQChannelNames.vi"() -> ("Number of \nExternal \nChannels 1"=w219:i32)  [unwired: 5 out]
      n131 = call "Auto Balance Error Tolerance DAO.vi"("Auto Balance Increment Actions"=w136, "LBCB Number"=w138) -> ("Auto Balance Error Out"=w217:T46)  [unwired: 3 in, 10 out]
      n132 = Build Array(w208, w166) -> (w167:T20[])
      n133 = call "Auto Balance Error Tolerance DAO.vi"("Auto Balance Increment Actions"=w136, "LBCB Number"=w137) -> ("Auto Balance Error Out"=w218:T46)  [unwired: 3 in, 10 out]
      n134 = Initialize Array(w119, 2 ("dimension size")) -> (w118:T5[])
      n135 = local write "Force Parameters"(w142) -> ()
      n136 = Build Array(w145, w144) -> (w143:T53[])
      n137 = Unbundle By Name(w154) -> ("Type"=w153:T52)
      n138 = Unbundle By Name(w155) -> ("Type"=w152:T52)
      n139 = local write "Number of \nExternal \nChannels"(w219) -> ()
      n140 = call "Actuator Point 2 Array.vi"("Actuator Point"=w217) -> ("Array"=w216:dbl[])
      n141 = call "Actuator Point 2 Array.vi"("Actuator Point"=w218) -> ("Array"=w168:dbl[])
      n142 = call "Load Previous Command.vi"("Number of LBCBs"=w209) -> ()  [unwired: 3 out]
      n143 = local write "Limits"(w167) -> ()
      n144 = local write "Target"(w118) -> ()
      n145 = local write "Force Groups"(w143) -> ()
      n146 = Build Array(w216, w168) -> (w169:dbl[][])
      n147 = local write "Auto Balance Error Tolerance"(w169) -> ()
      n148 = Build Array(w153, w152) -> (w151:T52[])
    }
  }
  n149 = Initialize Array(w23, w24) -> (w41:dbl[])
  n150 = Bundle By Name(cluster=T8 {"Displacements"=[], "Forces"=[], "Displacement \nCommands"=[]} ("element"), "Displacements"=w41, "Forces"=w41, "Displacement \nCommands"=w41) -> (w40:T8)
  n151 = Obtain Notifier(name (unnamed)="Mixed Mode Statuses", notification data type=w104, error in (no error)=w69) -> (notifier out=w105:refnum<notifier>, error out=w9:errorcluster)  [unwired: 1 in, 1 out]
  n152 = call "Create Archiving Transaction List.vi"("Volts Only"=w20, "Combined LBCBs"=w20, "Hold"=w18, "Number of LBCBs"=w17) -> ("Transactions"=w21:T30[])  [unwired: 7 in]
  n153 = Initialize Array(w23, w24, w24) -> (w22:dbl[][])
  n154 = call "Create Archiving Transaction List.vi"("Volts Only"=FALSE, "Combined LBCBs"=w13, "Hold"=w13, "Number of LBCBs"=Number_Of_LBCBs."2") -> ("Transactions"=w16:T30[])  [unwired: 7 in]
  n155 = call "Create Archiving Transaction List.vi"("Volts Only"=w18, "Combined LBCBs"=w20, "Hold"=w18, "Number of LBCBs"=w17) -> ("Transactions"=w19:T30[])  [unwired: 7 in]
  n156 = call "External Sensor Sensitivities DAO.vi"("Persistent DAO Actions"=Persistant_DAO_Actions."Get") -> ("Sensitivities Out"=w70:dbl[])  [unwired: 3 in, 7 out]
  n157 = Build Array(w40, w40) -> (w25:T8[])
  n158 = Obtain Queue(name (unnamed)="Parameter Changes", element data type=T42 {"Change State"=enum."Mixed Mode", "LBCB Number"=enum."LBCB1"} ("Parameter Changes"), error in (no error)=w9) -> (queue out=w113:refnum<queue>, error out=w91:errorcluster)  [unwired: 2 in, 1 out]
  n159 = while {
    shift-right: [w264] -> _
    shift-left: w25 -> [w263]
    tunnel: w70 -> [w294]
    shift-right: [w289] -> _
    shift-left: w105 -> [w290]
    tunnel: w104 -> [w288]
    tunnel: [w284] -> w96
    tunnel: w21 -> [w255]
    tunnel: w16 -> [w266]
    shift-right: [w265] -> _
    shift-left: w22 -> [w262]
    tunnel: T30[] [{"Dataset Source"=enum."External Sensors", "Dataset Type"=enum."LVDT", "Hold"=FALSE, "Volts"=TRUE, "Tag"=""}, {"Dataset Source"=enum."External Sensors", "Dataset Type"=enum."LVDT", "Hold"=FALSE, "Volts"=FALSE, "Tag"=""}] ("Transactions") -> [w253]
    shift-right: [w249] -> _
    shift-left: _ -> [w248]
    tunnel: w19 -> [w247]
    stop <- w284 stop-if-true
    w272 = 6 ("length")
    # "Ramp time times a multiplier loosely aligned\nwith Nyquist's rule of thumb"
    # "Status Changes Loop"
    n160 = local read "Cart Meas. Disp & Forces"() -> (w268:dbl[][])
    n161 = local read "External Sensors"() -> (w257:dbl[])
    n162 = local read "Measurements"() -> (w275:T23[])
    n163 = local read "Volts LVDT & LC"() -> (w273:dbl[][])
    n164 = local read "Averaging"() -> (w258:bool)
    n165 = local read "Servo Error"() -> (w269:dbl[][])
    n166 = local read "Commands"() -> (w260:T2[])
    n167 = local read "L2 Cmd  Volts"() -> (w274:dbl[])
    n168 = local read "L1 Cmd  Volts"() -> (w295:dbl[])
    n169 = local read "MixedModeStates"() -> (w280:T26)
    n170 = call "GetSamplingRate.vi"() -> ("Sampling"=w285:i32)
    n171 = Delete From Array(array=w273, length=w272, index (col)=w272) -> (deleted portion=w270:dbl[][], array with subset deleted=w271:dbl[][])  [unwired: 1 in]
    n172 = Multiply(x=w257, y=w294) -> (x*y=w259:dbl[])
    n173 = case shown="\"Update Command\"" w280 {
      tunnel: [FALSE TRUE TRUE TRUE TRUE TRUE TRUE TRUE TRUE TRUE TRUE TRUE] -> w276
      frame #0 {
      }
      frame #1 {
      }
      frame #2 {
      }
      frame #3 {
      }
      frame #4 {
      }
      frame #5 {
      }
      frame #6 {
      }
      frame #7 {
      }
      frame #8 {
      }
      frame #9 {
      }
      frame #10 {
      }
      frame #11 {
      }
    }
    n174 = local write "Status Changes"(w285) -> ()
    n175 = call "Sample Averaging.vi"("Sample In"=w259, "Averaging"=w258) -> ("Sample Out"=w250:dbl[])  [unwired: 9 in]
    n176 = local read "Rigid Connection"() -> (w245:bool)
    n177 = call "Average All.vi"("Rigid Connection"=w245, "Averaging"=w258, "Commands"=w260, "Individual Measurements"=w268, "Measurements"=w275) -> ("Data"=w246:dbl[][])  [unwired: 6 in]
    n178 = Build Array(w257, w250) -> (w254:dbl[][])
    n179 = Index Array(array=w253, index=1) -> (element=w251:T30)
    n180 = local read "Ramp Time"() -> (w293:u32)
    n181 = local read "Hold Period"() -> (w267:bool)
    n182 = call "Batch Dataset Store.vi"("Data"=w254, "Transactions"=w253) -> ()  [unwired: 9 in, 1 out]
    n183 = local read "Current Target"() -> (w279:T5[])
    n184 = local read "Iterative Target"() -> (w277:T5[])
    n185 = Multiply(x=w293, y=u32 2) -> (x*y=w291:u32)
    n186 = case shown="True" w267 {
      tunnel: w266 -> [_ w304]
      tunnel: [w298 w305] -> w265
      tunnel: w246 -> [_ w307]
      tunnel: [w299 w306] -> w264
      tunnel: w263 -> [w299 _]
      tunnel: w262 -> [w298 _]
      tunnel: w251 -> [_ w303]
      tunnel: w250 -> [_ w302]
      tunnel: [w297 w300] -> w249
      tunnel: w248 -> [w297 _]
      frame #0 {
      }
      frame #1 {
        n187 = call "Filter Hold Data.vi"("Data"=w307) -> ("Mixed Mode Data"=w306:T8[], "Hold Data"=w305:dbl[][])  [unwired: 9 in]
        n188 = call "Dataset.vi"("Dataset Trans Id"=w303, "Data In"=w302, "DAO Actions"=DAO_Actions."Set") -> ("Data Out"=w300:dbl[])  [unwired: 7 in, 1 out]
        n189 = call "Batch Dataset Store.vi"("Data"=w305, "Transactions"=w304) -> ()  [unwired: 9 in, 1 out]
      }
    }
    n190 = Wait Until Next ms Multiple(millisecond multiple=w291) -> ()  [unwired: 1 out]
    n191 = Build Array (concatenate)(w295, w274, w271, w270, w269) -> (w256:dbl[][])
    n192 = Select(t=w277, s=w276, f=w279) -> (s? t:f=w278:T5[])
    n193 = call "Filter Mixed Mode Data.vi"("Data"=w246) -> ("Mixed Mode Data"=w261:T14[])  [unwired: 10 in]
    n194 = local read "Convergence Status"() -> (w286:T25[])
    n195 = call "Batch Dataset Store.vi"("Data"=w246, "Transactions"=w247) -> ()  [unwired: 9 in, 1 out]
    n196 = call "Batch Dataset Store.vi"("Data"=w256, "Transactions"=w255) -> ()  [unwired: 9 in, 1 out]
    n197 = Bundle By Name(cluster=w288, "LBCB Target"=w278, "MixedModeStates"=w280, "LBCB Convergence"=w286, "LBCB Measurements"=w261) -> (w287:T40)
    n198 = local read "App Running"() -> (w296:bool)
    n199 = local read "L1 Autobalance Out"() -> (w283:T10[])
    n200 = local read "L2 Autobalance Out"() -> (w282:T10[])
    n201 = Not(x=w296) -> (.not. x?=w284:bool)
    n202 = local write "Hold Data"(w264) -> ()
    n203 = Send Notification(notification=w287, notifier=w290) -> (notifier out=w289:refnum<notifier>)  [unwired: 1 in, 1 out]
    n204 = call "Autobalance Data DAO.vi"("L2 Autobalance In"=w282, "L1 Autobalance Iin"=w283, "DAO Actions"=DAO_Actions."Set") -> ()  [unwired: 1 in, 8 out]
  }
  n205 = Flush Queue(queue=w113, error in (no error)=w91) -> (queue out=w92:refnum<queue>, error out=w90:errorcluster)  [unwired: 1 out]
  n206 = flat-sequence {
    tunnel: [w325] -> w75
    tunnel: [w327] -> w74
    tunnel: [w326] -> w73
    tunnel: w9 -> [_]
    tunnel: [w320] -> w67
    frame #0 {
      n207 = global read "Global Cache.vi" "L2 Calibrations"() -> (w328:T54)
      n208 = Unbundle By Name(w328) -> ("Command Sensitivity"=w325:dbl[], "Servo Error Offset"=w320:dbl[], "LVDT Sensitivity"=w322:dbl[], "LVDT Offset"=w324:dbl[], "Load Cell Offsets"=w323:dbl[], "Load Cell Sensitivity"=w321:dbl[])
      n209 = Build Array (concatenate)(w324, w323) -> (w327:dbl[])
      n210 = Build Array (concatenate)(w322, w321) -> (w326:dbl[])
    }
  }
  n211 = call "Init Mixed Mode Command.vi"("error in (no error)"=w9) -> ("error out"=w11:errorcluster, "Command Data"=w87:T5)  [unwired: 1 out]
  n212 = Initialize Array(0.0 ("Numeric"), 6 ("dimension size")) -> (w29:dbl[])
  n213 = Bundle By Name(cluster=T8 {"Displacements"=[], "Forces"=[], "Displacement \nCommands"=[]} ("element"), "Displacements"=w29, "Forces"=w29, "Displacement \nCommands"=w29) -> (w31:T8)
  n214 = Bundle By Name(cluster=w64, "Command"=Mixed_Mode_Command_Action."No Op", "Ramp Times"=cluster{"Initial":T38, "Iterative":T38} {"Initial"={"Ramp"=0.0, "Stab"=0.0, "Hold"=0.0}, "Iterative"={"Ramp"=0.0, "Stab"=0.0, "Hold"=0.0}}, "LBCB1"=w87, "LBCB2"=w87) -> (w86:T41)
  n215 = Obtain Queue(name (unnamed)="Mixed Mode Commands", element data type=w64, error in (no error)=w9) -> (queue out=w112:refnum<queue>, error out=w109:errorcluster)  [unwired: 2 in, 1 out]
  n216 = Bundle By Name(cluster=T34 {"Act Disp"=[], "Act Forces"=[], "Cart Disp"=[], "Cart Forces"=[]} ("Measurements Out"), "Act Disp"=w29, "Act Forces"=w29) -> (w30:T34)
  n217 = Flush Queue(queue=w112, error in (no error)=w109) -> (queue out=w63:refnum<queue>, error out=w6:errorcluster)  [unwired: 1 out]
  n218 = while {
    shift-right: [w340] -> _
    shift-left: w92 -> [w343]
    shift-right: [w332] -> _
    shift-left: w90 -> [w342]
    tunnel: [w336] -> w97
    tunnel: w66 -> [w335]
    tunnel: w46 -> [w334]
    tunnel: w64 -> [w331]
    shift-right: [w329] -> _
    shift-left: w63 -> [w330]
    stop <- w336 stop-if-true
    # "Parameter Changes Loop"
    n219 = Dequeue Element(queue=w343, timeout in ms (-1)=2000, error in (no error)=w342) -> (queue out=w340:refnum<queue>, element=w339:T42, timed out?=w341:bool, error out=w333:errorcluster)
    n220 = case shown="False" w341 {
      tunnel: w339 -> [w353 _]
      tunnel: w335 -> [w350 _]
      tunnel: w334 -> [w349 _]
      tunnel: w333 -> [w348 w542]
      tunnel: [w347 w542] -> w332
      tunnel: w331 -> [w346 _]
      tunnel: w330 -> [w345 w543]
      tunnel: [w344 w543] -> w329
      frame #0 {
        n221 = Unbundle By Name(w353) -> ("Change State"=w352:T43, "LBCB Number"=w351:T35)
        n222 = case shown="\"Stiffness Jacobian\"" w352 {
          tunnel: w351 -> [_ _ _ _ _ _ w480 _ w491 w502 w535 _]
          tunnel: w350 -> [_ _ _ _ w458 _ _ _ _ _ _ _]
          tunnel: w349 -> [_ _ _ _ _ _ _ _ _ w503 _ _]
          tunnel: w348 -> [w368 w391 w402 w406 w437 w461 w483 w487 w490 w500 w534 w540]
          tunnel: [w368 w391 w402 w406 w437 w461 w483 w487 w490 w499 w534 w540] -> w347
          tunnel: w346 -> [_ _ _ _ _ _ _ _ _ w498 _ _]
          tunnel: w345 -> [w367 w390 w401 w405 w436 w460 w482 w486 w489 w497 w533 w539]
          tunnel: [w367 w390 w401 w405 w436 w460 w482 w486 w489 w496 w533 w539] -> w344
          frame #0 {
            w358 = LBCB_Number."LBCB2" ("LBCB Number")
            w359 = LBCB_Number."LBCB1" ("LBCB Number")
            w360 = Persistant_DAO_Actions."Get" ("LBCB Settings Actions")
            n223 = call "Mixed Mode Force Error Range DAO.vi"("Force Error Range Actions"=w360, "LBCB Number"=w359) -> ("Force Error Range Out"=w377:T6)  [unwired: 3 in, 10 out]
            n224 = call "Mixed Mode Jacobian Gain DAO.vi"("Jacobian Gain Actions"=w360, "LBCB Number"=w359) -> ("Jacobian Gain Out"=w376:T6)  [unwired: 3 in, 10 out]
            n225 = call "Mixed Mode Max Increment DAO.vi"("Max Increment Actions"=w360, "LBCB Number"=w359) -> ("Max Increment Out"=w375:T6)  [unwired: 3 in, 10 out]
            n226 = call "Cartesian Point 2 Array.vi"("Cart Disp"=w375) -> ("Array"=w372:dbl[])  [unwired: 2 out]
            n227 = call "Cartesian Point 2 Array.vi"("Cart Disp"=w376) -> ("Array"=w373:dbl[])  [unwired: 2 out]
            n228 = call "Cartesian Point 2 Array.vi"("Cart Disp"=w377) -> ("Array"=w374:dbl[])  [unwired: 2 out]
            n229 = call "Mixed Mode Max Increment DAO.vi"("Max Increment Actions"=w360, "LBCB Number"=w358) -> ("Max Increment Out"=w369:T6)  [unwired: 3 in, 10 out]
            n230 = call "Mixed Mode Force Error Range DAO.vi"("Force Error Range Actions"=w360, "LBCB Number"=w358) -> ("Force Error Range Out"=w371:T6)  [unwired: 3 in, 10 out]
            n231 = call "Mixed Mode Jacobian Gain DAO.vi"("Jacobian Gain Actions"=w360, "LBCB Number"=w358) -> ("Jacobian Gain Out"=w370:T6)  [unwired: 3 in, 10 out]
            n232 = call "Cartesian Point 2 Array.vi"("Cart Disp"=w371) -> ("Array"=w365:dbl[])  [unwired: 1 in, 1 out]
            n233 = call "Cartesian Point 2 Array.vi"("Cart Disp"=w370) -> ("Array"=w363:dbl[])  [unwired: 1 in, 1 out]
            n234 = call "Cartesian Point 2 Array.vi"("Cart Disp"=w369) -> ("Array"=w361:dbl[])  [unwired: 1 in, 1 out]
            n235 = call "Force Control Parameters DAO.vi"("DAO Actions"=w360) -> ("Force Control Parameters Out"=w357:T9)  [unwired: 8 in, 2 out]
            n236 = call "Mixed Mode Force Group Priorities DAO.vi"("Force Error Range Actions"=w360, "LBCB Number"=w359) -> ("Force Group Priorities Out"=w356:T53)  [unwired: 11 in, 2 out]
            n237 = call "Mixed Mode Force Group Priorities DAO.vi"("Force Error Range Actions"=w360, "LBCB Number"=w358) -> ("Force Group Priorities Out"=w355:T53)  [unwired: 11 in, 2 out]
            n238 = Build Array(w356, w355) -> (w354:T53[])
            n239 = local write "Force Groups"(w354) -> ()
            n240 = Build Array(w374, w365) -> (w366:dbl[][])
            n241 = Build Array(w373, w363) -> (w364:dbl[][])
            n242 = Build Array(w372, w361) -> (w362:dbl[][])
            n243 = local write "Force Parameters"(w357) -> ()
            n244 = local write "Force Error Range"(w366) -> ()
            n245 = local write "Max Increment"(w362) -> ()
            n246 = local write "Jacobian Gain"(w364) -> ()
          }
          frame #1 {
            w386 = cluster{T24} {[[1000000.0, 0.0, 0.0, 0.0, 0.0, 0.0], [0.0, 1000000.0, 0.0, 0.0, 0.0, 0.0], [0.0, 0.0, 1000000.0, 0.0, 0.0, 0.0], [0.0, 0.0, 0.0, 1000000.0, 0.0, 0.0], [0.0, 0.0, 0.0, 0.0, 1000000.0, 0.0], [0.0, 0.0, 0.0, 0.0, 0.0, 1000000.0]]} ("Cluster")
            w379 = LBCB_Number."LBCB1" ("LBCB Number")
            w378 = LBCB_Number."LBCB2" ("LBCB Number")
            w380 = Persistant_DAO_Actions."Get" ("Actions")
            n247 = call "Stiffness Limits DAO.vi"("Cartesian Force Limit Actions"=w380, "ID"=w378) -> ("Stiffness Limit Out"=w383:T47)  [unwired: 11 in, 2 out]
            n248 = call "Stiffness Limits DAO.vi"("Cartesian Force Limit Actions"=w380, "ID"=w379) -> ("Stiffness Limit Out"=w385:T47)  [unwired: 11 in, 2 out]
            n249 = call "Stiffness Jacobian DAO.vi"("LBCB Number"=w379, "Actions"=w380) -> ("Stiffness Jacobian Out"=w393:T24)  [unwired: 3 in, 6 out]
            n250 = call "Stiffness Jacobian DAO.vi"("LBCB Number"=w378, "Actions"=w380) -> ("Stiffness Jacobian Out"=w392:T24)  [unwired: 3 in, 6 out]
            n251 = call "Actuator Matrix 2 2D Array.vi"("Matrix In"=w383) -> ("Matrix Out"=w382:T21)  [unwired: 10 out]
            n252 = call "Actuator Matrix 2 2D Array.vi"("Matrix In"=w385) -> ("Matrix Out"=w384:T21)  [unwired: 10 out]
            n253 = call "Calculated Stiffness Jacobian.vi"("Stiffness Jacobian In"=w393, "LBCB Number"=w379, "Actions"=w380) -> ()  [unwired: 1 in, 8 out]
            n254 = call "Calculated Stiffness Jacobian.vi"("Stiffness Jacobian In"=w392, "LBCB Number"=w378, "Actions"=w380) -> ()  [unwired: 1 in, 8 out]
            n255 = Build Array(w384, w382) -> (w381:dbl[][][])
            n256 = local write "Stiffness Limits"(w381) -> ()
            n257 = Bundle(cluster=w386, w392) -> (w387:cluster{T24})
            n258 = Bundle(cluster=w386, w393) -> (w389:cluster{T24})
            n259 = Build Array(w389, w387) -> (w388:cluster{T24}[])
            n260 = local write "Stiffness Jacobian"(w388) -> ()
          }
          frame #2 {
            w395 = Persistant_DAO_Actions."Get" ("Actions")
            n261 = call "LBCB Position DAO.vi"("LBCB Settings Actions"=w395, "LBCB Number"=LBCB_Number."LBCB1") -> ("LBCB Position Output"=w399:T22)  [unwired: 3 in, 10 out]
            n262 = call "LBCB Position DAO.vi"("LBCB Settings Actions"=w395, "LBCB Number"=LBCB_Number."LBCB2") -> ("LBCB Position Output"=w398:T22)  [unwired: 3 in, 10 out]
            n263 = call "Number Of LBCBs DAO.vi"("Actions"=w395) -> ("Rigid Connection Out"=w394:bool)  [unwired: 4 in, 6 out]
            n264 = local write "Rigid Connection"(w394) -> ()
            n265 = Build Array(w399, w398) -> (w400:T22[])
            n266 = local write "Position"(w400) -> ()
          }
          frame #3 {
            w408 = LBCB_Number."LBCB2" ("LBCB Number")
            w409 = LBCB_Number."LBCB1" ("LBCB Number")
            w407 = Persistant_DAO_Actions."Get" ("I Gain Actions")
            n267 = call "I Gain DAO.vi"("I Gain Actions"=w407, "LBCB Number"=w409) -> ("I Gain"=w418:T46)  [unwired: 3 in, 10 out]
            n268 = call "P Gain DAO.vi"("P Gain Actions"=w407, "LBCB Number"=w409) -> ("P Gain"=w417:T46)  [unwired: 3 in, 10 out]
            n269 = call "PID Controls DAO.vi"("Actions"=w407) -> ("PID Control  Out"=w414:T27)  [unwired: 3 in, 7 out]
            n270 = call "I Gain DAO.vi"("I Gain Actions"=w407, "LBCB Number"=w408) -> ("I Gain"=w412:T46)  [unwired: 3 in, 10 out]
            n271 = call "P Gain DAO.vi"("P Gain Actions"=w407, "LBCB Number"=w408) -> ("P Gain"=w413:T46)  [unwired: 3 in, 10 out]
            n272 = call "PID Controls DAO.vi"("Actions"=w407) -> ("PID Control  Out"=w403:T27)  [unwired: 3 in, 7 out]
            n273 = call "Actuator Point 2 Array.vi"("Actuator Point"=w418) -> ("Array"=w416:dbl[])
            n274 = call "Actuator Point 2 Array.vi"("Actuator Point"=w417) -> ("Array"=w415:dbl[])
            n275 = call "Actuator Point 2 Array.vi"("Actuator Point"=w412) -> ("Array"=w411:dbl[])
            n276 = call "Actuator Point 2 Array.vi"("Actuator Point"=w413) -> ("Array"=w410:dbl[])
            n277 = local write "L2 P Gain"(w410) -> ()
            n278 = local write "L2 I Gain"(w411) -> ()
            n279 = local write "L1 P Gain"(w415) -> ()
            n280 = local write "L1 I Gain"(w416) -> ()
            n281 = Build Array(w414, w403) -> (w404:T27[])
            n282 = local write "PID Control"(w404) -> ()
          }
          frame #4 {
            w428 = T2 {"Act Cmd"=[], "Cart Cmd"=[]} ("Data")
            w419 = LBCB_Number."LBCB2" ("ID")
            w421 = LBCB_Number."LBCB1" ("ID")
            w420 = Persistant_DAO_Actions."Get" ("Actuator Force Limit Actions")
            n283 = call "Command Voltage Limit DAO.vi"("Actuator Stroke Limit Actions"=w420, "ID"=w421) -> ("Command Voltage Limit Out"=w453:T45)  [unwired: 3 in, 10 out]
            n284 = call "Cartesian Increment Limits DAO.vi"("Actions"=w420, "LBCB Number"=w421) -> ("Inc Limits Out"=w430:T6)  [unwired: 11 in, 2 out]
            n285 = call "Actuator Force Limit DAO.vi"("Actuator Force Limit Actions"=w420, "ID"=w421) -> ("Actuator Force Limits Out"=w457:T45)  [unwired: 3 in, 10 out]
            n286 = call "Actuator Stroke Limit DAO.vi"("Actuator Stroke Limit Actions"=w420, "ID"=w421) -> ("Actuator Stroke Limits Out"=w456:T45)  [unwired: 3 in, 10 out]
            n287 = call "Cartesian Displacement Limit DAO.vi"("Cartesian Displacement Limit Actions"=w420, "ID"=w421) -> ("Cartesian Displacement Out"=w455:T47)  [unwired: 3 in, 10 out]
            n288 = call "Cartesian Force Limit DAO.vi"("Cartesian Force Limit Actions"=w420, "ID"=w421) -> ("Cartesian Force Limit Out"=w454:T47)  [unwired: 3 in, 10 out]
            n289 = call "Actuator Increment Limits DAO.vi"("Actions"=w420, "LBCB Number"=w421) -> ("Inc Limits Out"=w433:T46)  [unwired: 11 in, 2 out]
            n290 = call "Cartesian Point 2 Array.vi"("Cart Disp"=w430) -> ("Array"=w426:dbl[])  [unwired: 2 in]
            n291 = call "Cartesian Point 2 Array.vi"("Cart Disp"=w433) -> ("Array"=w427:dbl[])  [unwired: 2 in]
            n292 = call "Actuator Matrix 2 2D Array.vi"("Matrix In"=w453) -> ("Matrix Out"=w448:T21)  [unwired: 10 out]
            n293 = call "Cartesian Matrix 2 2D Array.vi"("Matrix In"=w455) -> ("Matrix Out"=w450:T21)  [unwired: 10 out]
            n294 = call "Actuator Matrix 2 2D Array.vi"("Matrix In"=w457) -> ("Matrix Out"=w452:T21)  [unwired: 10 out]
            n295 = call "Actuator Matrix 2 2D Array.vi"("Matrix In"=w456) -> ("Matrix Out"=w451:T21)  [unwired: 10 out]
            n296 = call "Cartesian Matrix 2 2D Array.vi"("Matrix In"=w454) -> ("Matrix Out"=w449:T21)  [unwired: 10 out]
            n297 = Bundle By Name(cluster=w458, "Actuator Force Limits"=w452, "Actuator Stroke Limits"=w451, "Cartesian Disp Limit"=w450, "Cartesian Force Limit"=w449, "Command Voltage Limit"=w448) -> (w459:T20)
            n298 = Bundle By Name(cluster=w428, "Act Cmd"=w427, "Cart Cmd"=w426) -> (w422:T2)
            n299 = call "Cartesian Increment Limits DAO.vi"("Actions"=w420, "LBCB Number"=w419) -> ("Inc Limits Out"=w429:T6)  [unwired: 11 in, 2 out]
            n300 = call "Actuator Increment Limits DAO.vi"("Actions"=w420, "LBCB Number"=w419) -> ("Inc Limits Out"=w432:T46)  [unwired: 11 in, 2 out]
            n301 = call "Command Voltage Limit DAO.vi"("Actuator Stroke Limit Actions"=w420, "ID"=w419) -> ("Command Voltage Limit Out"=w443:T45)  [unwired: 3 in, 10 out]
            n302 = call "Actuator Force Limit DAO.vi"("Actuator Force Limit Actions"=w420, "ID"=w419) -> ("Actuator Force Limits Out"=w447:T45)  [unwired: 3 in, 10 out]
            n303 = call "Actuator Stroke Limit DAO.vi"("Actuator Stroke Limit Actions"=w420, "ID"=w419) -> ("Actuator Stroke Limits Out"=w446:T45)  [unwired: 3 in, 10 out]
            n304 = call "Cartesian Displacement Limit DAO.vi"("Cartesian Displacement Limit Actions"=w420, "ID"=w419) -> ("Cartesian Displacement Out"=w445:T47)  [unwired: 3 in, 10 out]
            n305 = call "Cartesian Force Limit DAO.vi"("Cartesian Force Limit Actions"=w420, "ID"=w419) -> ("Cartesian Force Limit Out"=w444:T47)  [unwired: 3 in, 10 out]
            n306 = call "Cartesian Matrix 2 2D Array.vi"("Matrix In"=w444) -> ("Matrix Out"=w439:T21)  [unwired: 10 out]
            n307 = call "Cartesian Matrix 2 2D Array.vi"("Matrix In"=w445) -> ("Matrix Out"=w440:T21)  [unwired: 10 out]
            n308 = call "Cartesian Point 2 Array.vi"("Cart Disp"=w429) -> ("Array"=w424:dbl[])  [unwired: 2 in]
            n309 = call "Actuator Matrix 2 2D Array.vi"("Matrix In"=w443) -> ("Matrix Out"=w438:T21)  [unwired: 10 out]
            n310 = call "Actuator Matrix 2 2D Array.vi"("Matrix In"=w447) -> ("Matrix Out"=w442:T21)  [unwired: 10 out]
            n311 = call "Actuator Matrix 2 2D Array.vi"("Matrix In"=w446) -> ("Matrix Out"=w441:T21)  [unwired: 10 out]
            n312 = call "Cartesian Point 2 Array.vi"("Cart Disp"=w432) -> ("Array"=w425:dbl[])  [unwired: 2 in]
            n313 = Bundle By Name(cluster=w428, "Act Cmd"=w425, "Cart Cmd"=w424) -> (w423:T2)
            n314 = Bundle By Name(cluster=w458, "Actuator Force Limits"=w442, "Actuator Stroke Limits"=w441, "Cartesian Disp Limit"=w440, "Cartesian Force Limit"=w439, "Command Voltage Limit"=w438) -> (w434:T20)
            n315 = Build Array(w422, w423) -> (w431:T2[])
            n316 = Build Array(w459, w434) -> (w435:T20[])
            n317 = local write "Increment Limits"(w431) -> ()
            n318 = local write "Limits"(w435) -> ()
          }
          frame #5 {
            w462 = 1000.0 ("x")
            n319 = call "App Parameters DAO.vi"("Actions"=Persistant_DAO_Actions."Get") -> ("Application Timing and Logging Out"=w468:T48)  [unwired: 3 in, 7 out]
            n320 = Unbundle By Name(w468) -> ("Ramp Time.Interval"=w467:dbl, "Logging Directory"=w465:path, "Volt Logging Loop.Interval"=w464:dbl)
            n321 = Multiply(x=w462, y=w464) -> (x*y=w463:dbl)
            n322 = Multiply(x=w462, y=w467) -> (x*y=w466:dbl)
            n323 = local write "Volt Logger Time"(w463) -> ()
            n324 = local write "Logging Directory"(w465) -> ()
            n325 = local write "Ramp Time"(w466) -> ()
          }
          frame #6 {
            w473 = Persistant_DAO_Actions."Get" ("Auto Balance Increment Actions")
            n326 = case shown="\"LBCB2\"" w480 {
              tunnel: Control_Loop_State."Reset Autobalancing" ("L1 Ctrl Loop State") -> [w484 w485]
              frame #0 {
                n327 = local write "L1 Ctrl Loop State"(w484) -> ()
              }
              frame #1 {
                n328 = local write "L2 Ctrl Loop State"(w485) -> ()
              }
            }
            n329 = call "Autobalance Control DAO.vi"("Persistent DAO Actions"=Persistant_DAO_Actions."Get") -> ("Autobalance Control Out"=w478:T7)  [unwired: 8 in, 2 out]
            n330 = local write "AB Parameters"(w478) -> ()
            n331 = call "Auto Balance Error Tolerance DAO.vi"("Auto Balance Increment Actions"=w473, "LBCB Number"=LBCB_Number."LBCB1") -> ("Auto Balance Error Out"=w475:T46)  [unwired: 3 in, 10 out]
            n332 = call "Auto Balance Error Tolerance DAO.vi"("Auto Balance Increment Actions"=w473, "LBCB Number"=LBCB_Number."LBCB2") -> ("Auto Balance Error Out"=w472:T46)  [unwired: 3 in, 10 out]
            n333 = call "Actuator Point 2 Array.vi"("Actuator Point"=w475) -> ("Array"=w476:dbl[])
            n334 = call "Actuator Point 2 Array.vi"("Actuator Point"=w472) -> ("Array"=w470:dbl[])
            n335 = Build Array(w476, w470) -> (w477:dbl[][])
            n336 = local write "Auto Balance Error Tolerance"(w477) -> ()
          }
          frame #7 {
            n337 = local write "App Running"(FALSE ("App Running")) -> ()
          }
          frame #8 {
            n338 = case shown="\"LBCB1\"" w491 {
              tunnel: Control_Loop_State."Set Command" ("L1 Ctrl Loop State") -> [w493 w494]
              frame #0 {
                n339 = local write "L1 Ctrl Loop State"(w493) -> ()
              }
              frame #1 {
                n340 = local write "L2 Ctrl Loop State"(w494) -> ()
              }
            }
          }
          frame #9 {
            n341 = case shown="\"LBCB2\"" w502 {
              tunnel: Control_Loop_State."On" ("L1 Ctrl Loop State") -> [w531 w532]
              tunnel: [w531 w532] -> w495
              frame #0 {
                n342 = local write "L1 Ctrl Loop State"(w531) -> ()
              }
              frame #1 {
                n343 = local write "L2 Ctrl Loop State"(w532) -> ()
              }
            }
            n344 = case shown="\"2\"" w503 {
              tunnel: w502 -> [_ w513]
              tunnel: w495 -> [_ w512]
              tunnel: w500 -> [w505 w510]
              tunnel: [w505 w509] -> w499
              tunnel: w498 -> [_ w508]
              tunnel: w497 -> [w504 w507]
              tunnel: [w504 w506] -> w496
              frame #0 {
              }
              frame #1 {
                n345 = case shown="\"LBCB1\"" w513 {
                  tunnel: w512 -> [w526 w529]
                  tunnel: [w525 w528] -> w511
                  frame #0 {
                    n346 = local read "L2 Ctrl Loop State"() -> (w527:T15)
                    n347 = Equal?(x=w526, y=w527) -> (x = y?=w525:bool)
                  }
                  frame #1 {
                    n348 = local read "L1 Ctrl Loop State"() -> (w530:T15)
                    n349 = Equal?(x=w529, y=w530) -> (x = y?=w528:bool)
                  }
                }
                n350 = case shown="True" w511 {
                  tunnel: w510 -> [w515 w524]
                  tunnel: [w515 w523] -> w509
                  tunnel: w508 -> [_ w521]
                  tunnel: w507 -> [w514 w520]
                  tunnel: [w514 w519] -> w506
                  frame #0 {
                  }
                  frame #1 {
                    n351 = call "Persistant Ramp Time DAO.vi"("Ramp Time Actions"=Persistant_DAO_Actions."Get") -> ("Ramp Time Out"=w516:T56)  [unwired: 12 in, 2 out]
                    n352 = Bundle By Name(cluster=w521, "Command"=Mixed_Mode_Command_Action."Measure Initial Position", "Ramp Times"=w516) -> (w522:T41)
                    n353 = Enqueue Element(queue=w520, element=w522, error in (no error)=w524) -> (queue out=w519:refnum<queue>, error out=w523:errorcluster)  [unwired: 1 in, 1 out]
                  }
                }
              }
            }
          }
          frame #10 {
            n354 = case shown="\"LBCB1\"" w535 {
              tunnel: Control_Loop_State."Ready for Control" ("L1 Ctrl Loop State") -> [w537 w538]
              frame #0 {
                n355 = local write "L1 Ctrl Loop State"(w537) -> ()
              }
              frame #1 {
                n356 = local write "L2 Ctrl Loop State"(w538) -> ()
              }
            }
          }
          frame #11 {
            n357 = local write "DAQ Enabled"(TRUE ("DAQ Enabled")) -> ()
          }
        }
      }
      frame #1 {
        n358 = local read "L1 Ctrl Loop State"() -> (w549:T15)
        n359 = local read "L2 Ctrl Loop State"() -> (w546:T15)
        n360 = call "App Status Globals.vi"("App Status Actions"=App_Status_Actions."Get Status") -> ("App Status Out"=w553:T58)  [unwired: 5 in, 9 out]
        n361 = call "Control Loop State 2 Flags.vi"("L1 Ctrl Loop State"=w549) -> ("Controlled"=w547:bool, "Autobalanced"=w548:bool)
        n362 = local read "DAQ Started"() -> (w550:bool)
        n363 = call "Control Loop State 2 Flags.vi"("L1 Ctrl Loop State"=w546) -> ("Controlled"=w545:bool, "Autobalanced"=w544:bool)
        n364 = Bundle By Name(cluster=w553, "Controlling L2"=w545, "Autobalance L2"=w544, "Data Acquisition"=w550, "Controlling L1"=w547, "Autobalance L1"=w548) -> (w551:T58)
        n365 = call "App Status Globals.vi"("App Status Actions"=App_Status_Actions."Set All", "App Status In"=w551) -> ()  [unwired: 4 in, 10 out]
      }
    }
    n366 = local read "App Running"() -> (w338:bool)
    n367 = Not(x=w338) -> (.not. x?=w336:bool)
  }
  n368 = Obtain Queue(element data type=Command_or_Stiffness_Updates."Command Update" ("Command || Stiffness Update"), error in (no error)=w11) -> (queue out=w5:refnum<queue>, error out=w10:errorcluster)  [unwired: 3 in, 1 out]
  n369 = Initialize Array(0.0, 2 ("dimension size"), 6 ("dimension size")) -> (w34:dbl[][])
  n370 = Obtain Queue(name (unnamed)="Mixed Mode State", element data type=w111, error in (no error)=w10) -> (queue out=w101:refnum<queue>, error out=w108:errorcluster)  [unwired: 2 in, 1 out]
  n371 = Initialize Array(T16 {"Act Disp"={"X1"=TRUE, "X2"=TRUE, "Y1"=TRUE, "Z1"=TRUE, "Z2"=TRUE, "Z3"=TRUE}, "Act Force"={"X1"=TRUE, "X2"=TRUE, "Y1"=TRUE, "Z1"=TRUE, "Z2"=TRUE, "Z3"=TRUE}, "Act Incr"={"X1"=TRUE, "X2"=TRUE, "Y1"=TRUE, "Z1"=TRUE, "Z2"=TRUE, "Z3"=TRUE}, "Cart Disp"={"Dx"=TRUE, "Dy"=TRUE, "Dz"=TRUE, "Rx"=TRUE, "Ry"=TRUE, "Rz"=TRUE}, "Cart Force"={"Fx"=TRUE, "Fy"=TRUE, "Fz"=TRUE, "Mx"=TRUE, "My"=TRUE, "Mz"=TRUE}, "Cart Incr"={"Dx"=FALSE, "Dy"=FALSE, "Dz"=FALSE, "Rx"=FALSE, "Ry"=FALSE, "Rz"=FALSE}} ("Within Limits"), w44) -> (w48:T16[])
  n372 = Initialize Array(w31, w44) -> (w49:T8[])
  n373 = Initialize Array(w30, w44) -> (w50:T61)
  n374 = Build Array(LBCB_Number."LBCB1" ("LBCB Selected"), LBCB_Number."LBCB2" ("LBCB Selected")) -> (w59:T35[])
  n375 = while {
    shift-right: [w592] -> _
    shift-left: w111 -> [w584]
    shift-right: [w632] -> _
    shift-left: _ -> [w627]
    shift-right: [w630] -> _
    shift-left: u32 0 ("New Start Time") -> [w628]
    shift-right: [w626] -> _
    shift-left: w101 -> [w590]
    shift-right: [w621] -> _
    shift-left: w108 -> [w588]
    shift-right: [w585] -> _
    shift-left: w111 -> [w624]
    shift-right: [w622] -> _
    shift-left: w63 -> [w623]
    shift-right: [w618] -> _
    shift-left: w86 -> [w620]
    tunnel: [w615] -> w95
    tunnel: w46 -> [w614]
    shift-right: [w613] -> _
    shift-left: w50 -> [w578]
    shift-right: [w612] -> _
    shift-left: w43 -> [w576]
    shift-right: [w611] -> _
    shift-left: w49 -> [w608]
    tunnel: w59 -> [w575]
    shift-right: [w595] -> _
    shift-left: _ -> [w606]
    shift-right: [w596] -> _
    shift-left: _ -> [w605]
    shift-right: [w597] -> _
    shift-left: _ -> [w604]
    shift-right: [w593] -> _
    shift-left: w48 -> [w594]
    shift-right: [w583] -> _
    shift-left: w43 -> [w582]
    tunnel: w45 -> [w581]
    shift-right: [w574] -> _
    shift-left: _ -> [w573]
    shift-right: [w572] -> _
    shift-left: FALSE -> [w571]
    shift-right: [w558] -> _
    shift-left: w34 -> [w564]
    shift-right: [w557] -> _
    shift-left: w34 -> [w561]
    shift-right: [w555] -> _
    shift-left: w5 -> [w556]
    stop <- w615 stop-if-true
    # "Current Actuator\nPosition"
    # "Necessary because of \nthe PID loops"
    # "Make sure that overrides\nare broadcast and recorded"
    # "Needed for Convergence Check"
    # "Previous Hold Data"
    n376 = Unbundle By Name(w620) -> ("Command"=w619:T39)
    n377 = local read "Rigid Connection"() -> (w569:bool)
    n378 = local read "L1 Ctrl Loop Out Actuator"() -> (w562:dbl[])
    n379 = local read "L2 Ctrl Loop Out Actuator"() -> (w563:dbl[])
    n380 = case shown="\"Stop\"" w619 {
      tunnel: w584 -> [w1419 _ _ w1422 w1423 w1424]
      tunnel: [w1419 Mixed_Mode_States."Aborting" ("MixedModeStates") Mixed_Mode_States."Exit" ("MixedModeStates") w1422 w1423 w1424] -> w585
      frame #0 {
      }
      frame #1 {
      }
      frame #2 {
      }
      frame #3 {
      }
      frame #4 {
      }
      frame #5 {
      }
    }
    n381 = call "Current Position DAO.vi"("Rigid Connection"=w569, "Actions"=DAO_Actions."Get") -> ("LBCB 2 Commands Out"=w565:dbl[], "LBCB 1 Commands Out"=w566:dbl[])  [unwired: 8 in]
    n382 = local read "Position"() -> (w607:T22[])
    n383 = call "Ramp Timer.vi"("Previous Ramp Time"=w628) -> ("New Start Time"=w629:u32, "Current Ramp Time"=w631:u64)
    n384 = Replace Array Subset(array=w564, new element #1=w566, index (row) #1=0 ("index"), new element #2=w565, index (row) #2=1 ("index")) -> (w558:dbl[][])  [unwired: 2 in]
    n385 = Replace Array Subset(array=w561, new element #1=w562, index (row) #1=0 ("index (row)"), new element #2=w563, index (row) #2=1 ("index (row)")) -> (w557:dbl[][])  [unwired: 2 in]
    n386 = local read "Ramp Time"() -> (w609:u32)
    n387 = case shown="\"Start Initial Ramp\"" w585 {
      tunnel: [Mixed_Mode_States."Wait For DAQ" ("f") w859 Mixed_Mode_States."Idle" ("f") w909 Mixed_Mode_States."Initial Position" ("MixedModeStates") w950 w968 w1015 w1044 w1096 Mixed_Mode_States."Update Command" ("MixedModeStates") Mixed_Mode_States."Start Iterative Ramp" ("MixedModeStates") Mixed_Mode_States."Run Iterative Ramp" ("MixedModeStates") w1238 Mixed_Mode_States."Iterative Stabilize" ("MixedModeStates") w1275 Mixed_Mode_States."Iterative Holding" ("MixedModeStates") w1305 Mixed_Mode_States."Stabilize" ("MixedModeStates") w1335 Mixed_Mode_States."Holding" ("MixedModeStates") w1365 Mixed_Mode_States."Idle" ("f") Mixed_Mode_States."Exit" ("f") Mixed_Mode_States."Idle" ("f")] -> w591
      tunnel: [T38 {"Ramp"=0.0, "Stab"=0.0, "Hold"=0.0} ("Initial") w861 w893 w913 w920 w947 w974 w1034 w1064 w1107 w1145 w1191 w1229 w1251 w1270 w1284 w1301 w1319 w1330 w1344 w1361 w1379 w1392 w1399 w1411] -> w632
      tunnel: w631 -> [_ _ _ _ _ w944 _ w1018 _ _ _ _ _ w1253 _ w1286 _ w1316 _ w1346 _ w1376 _ _ _]
      tunnel: [w837 w860 w892 w912 w923 w951 w982 w1035 w1062 w1106 w1144 w1190 w1230 w1252 w1271 w1292 w1300 w1322 w1331 w1352 w1360 w1382 w1391 w1401 w1409] -> w630
      tunnel: w629 -> [_ _ _ _ w923 _ w982 _ _ _ _ _ w1230 _ w1271 _ w1300 _ w1331 _ w1360 _ _ _ _]
      tunnel: w628 -> [w837 w860 w892 w912 _ w951 _ w1035 w1062 w1106 w1144 w1190 _ w1252 _ w1292 _ w1322 _ w1352 _ w1382 w1391 w1401 w1409]
      tunnel: w627 -> [_ w861 w893 w913 _ w947 _ w1034 w1064 w1107 w1145 w1191 _ w1251 _ w1284 w1301 w1319 _ w1344 w1361 w1379 w1392 w1399 w1411]
      tunnel: w619 -> [_ w848 _ w910 _ _ _ _ _ _ _ _ _ _ _ _ _ _ _ _ _ _ _ _ _]
      tunnel: w624 -> [_ _ _ _ _ _ _ _ _ _ _ _ _ _ _ _ _ _ _ _ _ _ _ _ _]
      tunnel: w623 -> [w834 w857 w889 w905 w922 w940 w978 w1029 w1061 w1102 w1142 w1188 w1224 w1248 w1269 w1281 w1298 w1311 w1329 w1341 w1359 w1371 w1389 w1397 w1408]
      tunnel: [w834 w856 w889 w904 w922 w939 w978 w1028 w1061 w1102 w1142 w1188 w1224 w1247 w1269 w1280 w1298 w1310 w1329 w1340 w1359 w1370 w1389 w1397 w1408] -> w622
      tunnel: [w832 w855 w887 w903 w919 w937 w977 w1026 w1060 w1101 w1143 w1187 w1223 w1245 w1268 w1278 w1299 w1308 w1328 w1338 w1358 w1368 w1390 w1398 w1407] -> w618
      tunnel: w620 -> [w833 w852 w888 w900 w921 w938 w975 w1027 w1060 w1101 w1143 w1187 w1223 w1246 w1268 w1279 w1299 w1309 w1328 w1339 w1358 w1369 w1390 w1398 w1407]
      tunnel: [_ _ _ _ _ w930 _ w1032 _ _ _ _ _ w1240 _ _ _ _ _ _ _ _ _ _ _] -> w610
      tunnel: w607 -> [_ _ w884 _ _ w932 _ w1024 _ _ _ _ _ w1241 _ _ _ _ _ _ _ _ _ _ _]
      tunnel: w614 -> [_ _ w886 _ _ w933 _ w1025 _ _ _ _ _ w1244 _ _ _ _ _ _ _ _ _ _ _]
      tunnel: [w825 w843 w883 w897 w915 w935 w965 w1022 w1055 w1094 w1137 w1178 w1222 w1239 w1267 w1276 w1297 w1306 w1327 w1336 w1357 w1366 w1388 w1396 w1405] -> w580
      tunnel: w581 -> [_ _ w885 _ _ w934 _ w1023 _ _ _ _ _ w1242 _ _ _ _ _ _ _ _ _ _ _]
      tunnel: w609 -> [_ w846 w879 w899 _ w936 _ w1021 _ _ _ _ _ w1243 _ w1277 _ w1307 _ w1337 _ w1367 w1386 _ _]
      tunnel: w575 -> [_ _ _ _ _ _ _ _ w1056 w1084 _ w1182 _ _ _ _ _ _ _ _ _ _ _ _ _]
      tunnel: w608 -> [_ _ _ _ _ _ _ _ _ _ w1139 _ _ _ _ _ _ _ _ _ _ _ _ _ _]
      tunnel: w569 -> [_ _ w866 _ _ w926 _ w1014 _ _ _ _ _ w1237 _ _ _ _ _ _ _ _ _ _ _]
      tunnel: [w824 w842 w878 w896 w917 w929 w964 w1013 w1051 w1087 w1133 w1175 w1220 w1236 w1265 w1274 w1295 w1304 w1325 w1334 w1355 w1364 w1385 w1395 w1404] -> w574
      tunnel: w573 -> [w824 w842 w878 w896 w917 w929 w964 w1013 _ w1087 w1133 w1175 w1220 w1236 w1265 w1274 w1295 w1304 w1325 w1334 w1355 w1364 w1385 w1395 w1404]
      tunnel: [w823 w841 w877 w895 w916 w928 w963 w1012 FALSE w1086 w1132 TRUE w1219 w1235 w1264 w1273 w1294 w1303 w1324 w1333 w1354 w1363 w1384 w1394 w1403] -> w572
      tunnel: w571 -> [w823 w841 w877 w895 w916 w928 w963 w1012 _ w1086 w1132 _ w1219 w1235 w1264 w1273 w1294 w1303 w1324 w1333 w1354 w1363 w1384 w1394 w1403]
      tunnel: w557 -> [_ _ w869 _ _ w927 _ _ _ _ _ _ _ _ _ _ _ _ _ _ _ _ _ _ _]
      tunnel: w558 -> [_ _ _ _ _ _ w962 w1011 _ _ _ w1173 _ w1234 _ _ _ _ _ _ _ _ _ _ _]
      tunnel: w556 -> [w822 w840 w865 w894 w914 w925 w960 w1009 w1046 w1083 w1128 w1172 w1217 w1232 w1263 w1272 w1293 w1302 w1323 w1332 w1353 w1362 w1383 w1393 w1402]
      tunnel: [w822 w840 w865 w894 w914 w925 w959 w1009 w1045 w1083 w1127 w1172 w1216 w1232 w1263 w1272 w1293 w1302 w1323 w1332 w1353 w1362 w1383 w1393 w1402] -> w555
      frame #0 {
        n388 = call "Init Mixed Mode Command.vi"() -> ("Command Data"=w829:T5)  [unwired: 1 in, 2 out]
        n389 = Build Array(MM_Result_Actions."Nop" ("MM Result Actions")) -> (w825:T1[])
        n390 = call "Mixed Mode Commands DAO.vi"("Mixed Mode Commands\n Datastore Actions"=DAO_Actions."Init" ("Mixed Mode Commands\n Datastore Actions")) -> ()  [unwired: 3 in, 8 out]
        n391 = Bundle By Name(cluster=w833, "Command"=Mixed_Mode_Command_Action."No Op", "Ramp Times"=cluster{"Initial":T38, "Iterative":T38} {"Initial"={"Ramp"=0.0, "Stab"=0.0, "Hold"=0.0}, "Iterative"={"Ramp"=0.0, "Stab"=0.0, "Hold"=0.0}}, "LBCB1"=w829, "LBCB2"=w829) -> (w832:T41)
        n392 = call "Stiffness Jacobian DAO.vi"("LBCB Number"=LBCB_Number."LBCB1" ("LBCB Selected"), "Actions"=Persistant_DAO_Actions."Init" ("Stiffness Jacobian Datastore Actions")) -> ()  [unwired: 3 in, 7 out]
        n393 = call "Convergence Status DAO.vi"("Actions"=Persistant_DAO_Actions."Init") -> ()  [unwired: 3 in, 8 out]
      }
      frame #1 {
        w843 = T1[] [enum."Check Limits"] items=["Nop", "Set Command", "Check Limits", "Send Command", "Store Prev Reading", "Averaging On", "Averaging Off", "Hold On", "Hold Off", "PID Hold On", "PID Hold Off", "Clear Increment Faults", "Set Initial Position"]
        n394 = Equal?(x=w848, y=Mixed_Mode_Command_Action."Measure Initial Position") -> (x = y?=w845:bool)
        n395 = Dequeue Element(queue=w857, timeout in ms (-1)=w846) -> (queue out=w856:refnum<queue>, element=w853:T41, timed out?=w854:bool)  [unwired: 1 in, 1 out]
        n396 = Select(t=Mixed_Mode_States."Start Initial Position", s=w845, f=Mixed_Mode_States."Idle" ("MixedModeStates")) -> (s? t:f=w849:T26)
        n397 = Equal?(x=Mixed_Mode_Command_Action."Start Command", y=w848) -> (x = y?=w844:bool)
        n398 = Select(t=w852, s=w854, f=w853) -> (s? t:f=w855:T41)
        n399 = case shown="True" w844 {
          tunnel: [w862 Mixed_Mode_States."Start Initial Ramp" ("MixedModeStates")] -> w859
          tunnel: w849 -> [w862 _]
          frame #0 {
          }
          frame #1 {
            n400 = call "Ramp Time DAO.vi"("Actions"=DAO_Actions."Init") -> ()  [unwired: 8 in, 3 out]
          }
        }
      }
      frame #2 {
        w883 = T1[] [enum."Averaging Off", enum."Hold Off", enum."PID Hold Off"] items=["Nop", "Set Command", "Check Limits", "Send Command", "Store Prev Reading", "Averaging On", "Averaging Off", "Hold On", "Hold Off", "PID Hold On", "PID Hold Off", "Clear Increment Faults", "Set Initial Position"]
        n401 = Wait Until Next ms Multiple(millisecond multiple=w879) -> ()  [unwired: 1 out]
        n402 = call "Cntrl Loop Actuator Out 2 MM Comand.vi"("Act Cmds In"=w869, "Number of\nLBCBs In"=w886, "LBCB Type"=w885, "Position"=w884) -> ("Cmd Out"=w868:T2[])  [unwired: 11 in]
        n403 = call "Rigid Connection Command Reverse Filter.vi"("Rigid Connection"=w866, "LBCB Commands In"=w868) -> ("LBCB Commands Out"=w867:T2[])  [unwired: 9 in]
        n404 = call "Initial Target.vi"("Initial Position"=w867) -> ("Initial Target"=w881:T5[])
        n405 = Index Array(array=w868, index #1=0 ("index"), index #2=1 ("index")) -> (element #1=w873:T2, element #2=w872:T2)
        n406 = Bundle By Name(cluster=w888, "Command"=Mixed_Mode_Command_Action."No Op") -> (w887:T41)
        n407 = Unbundle By Name(w872) -> ("Cart Cmd"=w870:dbl[])
        n408 = Unbundle By Name(w873) -> ("Cart Cmd"=w871:dbl[])
        n409 = call "Mixed Mode Commands DAO.vi"("Current Target In"=w881, "Mixed Mode Commands\n Datastore Actions"=DAO_Actions."Set" ("Mixed Mode Commands\n Datastore Actions")) -> ("Current Target"=w880:T5[])  [unwired: 7 in, 2 out]
        n410 = local write "Current Target"(w880) -> ()
        n411 = call "Current Position DAO.vi"("Rigid Connection"=w866, "LBCB 2 Commands In"=w870, "LBCB 1 Commands In"=w871, "Actions"=DAO_Actions."Set") -> ()  [unwired: 6 in, 2 out]
      }
      frame #3 {
        n412 = Build Array(MM_Result_Actions."Nop" ("MM Result Actions")) -> (w897:T1[])
        n413 = Dequeue Element(queue=w905, timeout in ms (-1)=w899) -> (queue out=w904:refnum<queue>, element=w901:T41, timed out?=w902:bool)  [unwired: 1 in, 1 out]
        n414 = Select(t=w900, s=w902, f=w901) -> (s? t:f=w903:T41)
        n415 = Equal?(x=Mixed_Mode_Command_Action."Start Acquisition", y=w910) -> (x = y?=w906:bool)
        n416 = Select(t=Mixed_Mode_States."Idle" ("MixedModeStates"), s=w906, f=Mixed_Mode_States."Wait For DAQ" ("MixedModeStates")) -> (s? t:f=w909:T26)
      }
      frame #4 {
        w915 = T1[] [enum."Averaging On", enum."Hold On"] items=["Nop", "Set Command", "Check Limits", "Send Command", "Store Prev Reading", "Averaging On", "Averaging Off", "Hold On", "Hold Off", "PID Hold On", "PID Hold Off", "Clear Increment Faults", "Set Initial Position"]
        n417 = Unbundle By Name(w921) -> ("Ramp Times.Initial"=w920:T38)
        n418 = Bundle By Name(cluster=w921, "Command"=Mixed_Mode_Command_Action."No Op") -> (w919:T41)
      }
      frame #5 {
        w935 = T1[] [enum."Averaging On", enum."Hold On", enum."Set Initial Position", enum."Check Limits"] items=["Nop", "Set Command", "Check Limits", "Send Command", "Store Prev Reading", "Averaging On", "Averaging Off", "Hold On", "Hold Off", "PID Hold On", "PID Hold Off", "Clear Increment Faults", "Set Initial Position"]
        n419 = Unbundle By Name(w947) -> ("Hold"=w943:dbl)
        n420 = Divide(x=w944, y=u64 1000) -> (x/y=w946:dbl)
        n421 = Greater?(x=w946, y=w943) -> (0:w931:bool)
        n422 = Dequeue Element(queue=w940, timeout in ms (-1)=w936) -> (queue out=w939:refnum<queue>, element=w941:T41, timed out?=w942:bool)  [unwired: 1 in, 1 out]
        n423 = call "Cntrl Loop Actuator Out 2 MM Comand.vi"("Act Cmds In"=w927, "Number of\nLBCBs In"=w933, "LBCB Type"=w934, "Position"=w932) -> ("Cmd Out"=w930:T2[])  [unwired: 11 in]
        n424 = case shown="True" w931 {
          tunnel: w930 -> [_ w955]
          tunnel: w926 -> [_ w953]
          frame #0 {
          }
          frame #1 {
            w957 = DAO_Actions."Set" ("Mixed Mode Commands\n Datastore Actions")
            n425 = call "Rigid Connection Command Reverse Filter.vi"("Rigid Connection"=w953, "LBCB Commands In"=w955) -> ("LBCB Commands Out"=w954:T2[])  [unwired: 9 in]
            n426 = call "Commands 2 Cart Commands.vi"("Cmd In"=w955) -> ("Cart Commands Out"=w956:dbl[][])  [unwired: 10 in]
            n427 = call "Initial Target.vi"("Initial Position"=w954) -> ("Initial Target"=w958:T5[])
            n428 = call "Start Position DAO.vi"("Displacements In"=w956, "DAO Actions"=w957) -> ()  [unwired: 8 in, 2 out]
            n429 = call "Mixed Mode Commands DAO.vi"("Current Target In"=w958, "Mixed Mode Commands\n Datastore Actions"=w957) -> ("Current Target"=w952:T5[])  [unwired: 7 in, 2 out]
            n430 = local write "Current Target"(w952) -> ()
            n431 = local write "Target"(w952) -> ()
          }
        }
        n432 = Select(t=w938, s=w942, f=w941) -> (s? t:f=w937:T41)
        n433 = Select(t=Mixed_Mode_States."Done" ("MixedModeStates"), s=w931, f=Mixed_Mode_States."Initial Position") -> (s? t:f=w950:T26)
      }
      frame #6 {
        w965 = T1[] [enum."Clear Increment Faults"] items=["Nop", "Set Command", "Check Limits", "Send Command", "Store Prev Reading", "Averaging On", "Averaging Off", "Hold On", "Hold Off", "PID Hold On", "PID Hold Off", "Clear Increment Faults", "Set Initial Position"]
        # "The idea is that the initial position is fed into the target DAO and maintained for\nall DOFs that are not being commanded for displacement"
        n434 = Unbundle By Name(w975) -> ("Ramp Times.Initial"=w974:T38, "LBCB1"=w973:T5, "LBCB2"=w970:T5)
        n435 = Build Array(w973, w970) -> (w967:T5[])
        n436 = for {
          tunnel: w967 -> [w993] mode=indexing
          tunnel: [w995] -> w971 mode=indexing
          tunnel: w962 -> [w992] mode=indexing
          tunnel: [w990] -> w966 mode=indexing
          n437 = Unbundle By Name(w993) -> ("Command Type"=w996:enum16{"<None>", "Displacement", "Force"}[], "Displacements"=w994:dbl[])
          n438 = for {
            tunnel: w996 -> [w1001] mode=indexing
            tunnel: [w1003] -> w995 mode=indexing
            tunnel: w992 -> [w998] mode=indexing
            shift-right: [w997] -> w991
            shift-left: w994 -> [w1000]
            i -> [w999]
            n439 = case shown="\"Displacement\"" w1001 {
              tunnel: w1000 -> [w1004 w1008]
              tunnel: [w1004 w1005] -> w997
              tunnel: w999 -> [_ w1007]
              tunnel: w998 -> [_ w1006]
              frame #0 {
              }
              frame #1 {
                # "Add Current\nDisp for Force\nControl"
                n440 = Replace Array Subset(array=w1008, new element=w1006, index=w1007) -> (w1005:dbl[])
              }
            }
            n441 = Equal?(x=enum16{"<None>", "Displacement", "Force"}."Displacement", y=w1001) -> (x = y?=w1003:bool)
          }
          n442 = Bundle By Name(cluster=w993, "Displacements"=w991) -> (w990:T5)
        }
        n443 = Unbundle By Name(w974) -> ("Ramp"=w985:dbl)
        n444 = Equal To 0?(x=w985) -> (x = 0?=w984:bool)
        n445 = Or Array Elements(Boolean array=w971) -> (logical OR=w961:bool)
        n446 = case shown="False" w961 {
          tunnel: w960 -> [w986 w989]
          tunnel: [w986 w987] -> w959
          frame #0 {
          }
          frame #1 {
            n447 = Enqueue Element(queue=w989, element=Command_or_Stiffness_Updates."Command Update") -> (queue out=w987:refnum<queue>)  [unwired: 2 in, 2 out]
          }
        }
        n448 = call "Mixed Mode Commands DAO.vi"("Current Target In"=w966, "Mixed Mode Commands\n Datastore Actions"=DAO_Actions."Set" ("Mixed Mode Commands\n Datastore Actions")) -> ("Current Target"=w969:T5[])  [unwired: 3 in, 6 out]
        n449 = local write "Current Target"(w969) -> ()
        n450 = Bundle By Name(cluster=w975, "Command"=Mixed_Mode_Command_Action."No Op") -> (w977:T41)
        n451 = Select(t=Mixed_Mode_States."Run Initial Ramp" ("MixedModeStates"), s=w961, f=Mixed_Mode_States."Start Iterative Stage" ("MixedModeStates")) -> (s? t:f=w981:T26)
        n452 = Select(t=Mixed_Mode_States."Idle" ("MixedModeStates"), s=w984, f=w981) -> (s? t:f=w968:T26)
      }
      frame #7 {
        w1022 = T1[] [enum."Set Command", enum."Check Limits", enum."Send Command"] items=["Nop", "Set Command", "Check Limits", "Send Command", "Store Prev Reading", "Averaging On", "Averaging Off", "Hold On", "Hold Off", "PID Hold On", "PID Hold Off", "Clear Increment Faults", "Set Initial Position"]
        n453 = call "Ramp Time DAO.vi"("Actions"=DAO_Actions."Get") -> ("Ramp Time Out"=w1019:u64)  [unwired: 8 in, 2 out]
        n454 = Add(x=w1019, y=w1018) -> (x+y=w1017:u64)
        n455 = call "Ramp Time Completions.vi"("Current Ramp Time"=w1017, "Initial"=w1034) -> ("Still in Ramp"=w1016:bool, "Fraction\nCompleted"=w1033:dbl)
        n456 = case shown="True" w1016 {
          tunnel: w1033 -> [w1038 _]
          tunnel: [Mixed_Mode_States."Run Initial Ramp" ("MixedModeStates") Mixed_Mode_States."Start Iterative Stage" ("MixedModeStates")] -> w1015
          tunnel: [w1036 w1040] -> w1010
          frame #0 {
            n457 = call "Calculate Ramp Displacements.vi"("Ramp Time"=w1038) -> ("Target"=w1036:T5[])  [unwired: 2 in]
          }
          frame #1 {
            n458 = call "Mixed Mode Commands DAO.vi"("Mixed Mode Commands\n Datastore Actions"=DAO_Actions."Get" ("Mixed Mode Commands\n Datastore Actions")) -> ("Current Target"=w1040:T5[])  [unwired: 3 in, 7 out]
          }
        }
        n459 = Dequeue Element(queue=w1029, timeout in ms (-1)=w1021) -> (queue out=w1028:refnum<queue>, element=w1031:T41, timed out?=w1030:bool)  [unwired: 1 in, 1 out]
        n460 = Select(t=w1027, s=w1030, f=w1031) -> (s? t:f=w1026:T41)
        n461 = local write "Target"(w1010) -> ()
        n462 = call "MM Command to Cntrl Loop Actuator In.vi"("Target"=w1010, "Current Cartesian Position"=w1011, "Number of\nLBCBs In"=w1025, "LBCB Type"=w1023, "Position"=w1024, "Rigid Connection"=w1014) -> ("Cmd Out"=w1032:T2[])  [unwired: 5 in, 4 out]
      }
      frame #8 {
        w1055 = T1[] [enum."Check Limits", enum."Store Prev Reading"] items=["Nop", "Set Command", "Check Limits", "Send Command", "Store Prev Reading", "Averaging On", "Averaging Off", "Hold On", "Hold Off", "PID Hold On", "PID Hold Off", "Clear Increment Faults", "Set Initial Position"]
        # "Store Force Parameters for \nthis cycle of force ramps"
        # "Initialize the Multi DOF State Machine"
        # "Transfer Current Displacement to the Force Target"
        n463 = Unbundle By Name(w1060) -> ("LBCB1"=w1059:T5, "LBCB2"=w1057:T5)
        n464 = Build Array(w1059, w1057) -> (w1058:T5[])
        n465 = for {
          tunnel: T25 {"IsConverged"=[], "Force Errors"=[], "Controlling DOF"=[]} ("Convergence Status Out") -> [w1078]
          tunnel: w1058 -> [w1073] mode=indexing
          tunnel: [w1071] -> w1053 mode=indexing
          tunnel: w1056 -> [w1070] mode=indexing
          tunnel: [w1069] -> w1047 mode=indexing
          n466 = Unbundle By Name(w1073) -> ("Command Type"=w1079:enum16{"<None>", "Displacement", "Force"}[])
          n467 = for {
            tunnel: w1079 -> [w1080] mode=indexing
            tunnel: [w1082] -> w1069 mode=indexing
            n468 = Not Equal?(x=enum16{"<None>", "Displacement", "Force"}."Force", y=w1080) -> (x != y?=w1082:bool)
          }
          n469 = Initialize Array(0.0 ("element"), 6 ("dimension size")) -> (w1074:dbl[])
          n470 = Bundle By Name(cluster=w1078, "IsConverged"=w1069, "Force Errors"=w1074) -> (w1077:T25)
          n471 = call "Convergence Status DAO.vi"("Convergence Status In"=w1077, "LBCB Selected"=w1070, "Actions"=Persistant_DAO_Actions."Set") -> ("Convergence Status Out"=w1071:T25)  [unwired: 1 in, 7 out]
        }
        n472 = Or Array Elements(Boolean array=w1047) -> (logical OR=w1043:bool)
        n473 = local read "Force Parameters"() -> (w1051:T9)
        n474 = case shown="False" w1043 {
          tunnel: w1046 -> [w1067 w1068]
          tunnel: [w1065 w1068] -> w1045
          frame #0 {
            n475 = Enqueue Element(queue=w1067, element=Command_or_Stiffness_Updates."Command Update") -> (queue out=w1065:refnum<queue>)  [unwired: 2 in, 2 out]
          }
          frame #1 {
          }
        }
        n476 = call "MM Multi DOF Status DAO.vi"("Actions"=DAO_Actions."Init") -> ("error out"=w1049:errorcluster)  [unwired: 9 in, 1 out]
        n477 = call "MM Multi DOF State Machine.vi"("error in (no error)"=w1049, "Force Control Parameters"=w1051, "Convergence Status In"=w1053) -> ("Convergence Status Out"=w1052:T25[])  [unwired: 7 in, 1 out]
        n478 = local write "Convergence Status"(w1052) -> ()
        n479 = Select(t=Mixed_Mode_States."Start Hold", s=w1043, f=Mixed_Mode_States."Start Iterative Stabilize" ("MixedModeStates")) -> (s? t:f=w1044:T26)
      }
      frame #9 {
        w1094 = T1[] [enum."Hold Off", enum."Averaging Off"] items=["Nop", "Set Command", "Check Limits", "Send Command", "Store Prev Reading", "Averaging On", "Averaging Off", "Hold On", "Hold Off", "PID Hold On", "PID Hold Off", "Clear Increment Faults", "Set Initial Position"]
        n480 = local read "Hold Data"() -> (w1095:T8[])
        n481 = call "Mixed Mode Commands DAO.vi"("Mixed Mode Commands\n Datastore Actions"=DAO_Actions."Get" ("Mixed Mode Commands\n Datastore Actions")) -> ("Current Target"=w1099:T5[])  [unwired: 3 in, 7 out]
        n482 = Unbundle By Name(w1087) -> ("Multi Command Update"=w1097:bool)
        n483 = Not(x=w1086) -> (.not. x?=w1085:bool)
        n484 = local read "Force Error Range"() -> (w1093:dbl[][])
        n485 = for {
          tunnel: [w1120] -> w1089 mode=indexing
          tunnel: w1093 -> [w1122] mode=indexing
          tunnel: w1099 -> [w1125] mode=indexing
          tunnel: w1095 -> [w1124] mode=indexing
          tunnel: w1084 -> [w1119] mode=indexing
          n486 = Unbundle By Name(w1124) -> ("Forces"=w1123:dbl[])
          n487 = call "Convergence Status DAO.vi"("LBCB Selected"=w1119, "Actions"=DAO_Actions."Get") -> ("Convergence Status Out"=w1126:T25)  [unwired: 2 in, 7 out]
          n488 = call "Convergence Check.vi"("Forces Error \nTolerances"=w1122, "Command Data"=w1125, "Cart\nForces"=w1123, "Mixed Mode Convergence Status In"=w1126) -> ("Mixed Mode Convergence Status Out"=w1120:T25)  [unwired: 2 in, 5 out]
        }
        n489 = local read "Force Groups"() -> (w1092:T6[])
        n490 = Or(x=w1085, y=w1097) -> (x .or. y?=w1098:bool)
        n491 = call "MM Multi DOF State Machine.vi"("Force Control Parameters"=w1087, "Convergence Status In"=w1089) -> ("Convergence Status Out"=w1088:T25[])  [unwired: 8 in, 1 out]
        n492 = for {
          tunnel: w1093 -> [w1116] mode=indexing
          tunnel: w1092 -> [w1115] mode=indexing
          tunnel: w1088 -> [w1114] mode=indexing
          tunnel: w1084 -> [w1110] mode=indexing
          tunnel: [w1113] -> w1091 mode=indexing
          tunnel: [w1112] -> w1090 mode=indexing
          tunnel: w1087 -> [w1111]
          n493 = call "Pick A DOF.vi"("LBCB Number"=w1110, "Force Control Parameters"=w1111, "Force Group Priorities"=w1115, "Forces Error \nWindow"=w1116, "Mixed Mode Convergence Status In"=w1114) -> ("Mixed Mode Convergence Status Out"=w1118:T25)  [unwired: 5 in, 1 out]
          n494 = Unbundle By Name(w1118) -> ("IsConverged"=w1113:bool[])
          n495 = call "Convergence Status DAO.vi"("Convergence Status In"=w1118, "LBCB Selected"=w1110, "Actions"=DAO_Actions."Set") -> ("Convergence Status Out"=w1112:T25)  [unwired: 1 in, 7 out]
        }
        n496 = Select(t=Mixed_Mode_States."Update Command", s=w1098, f=Mixed_Mode_States."Update Stiffness Jacobian") -> (s? t:f=w1104:T26)
        n497 = And Array Elements(Boolean array=w1091) -> (logical AND=w1109:bool)
        n498 = local write "Convergence Status"(w1090) -> ()
        n499 = Select(t=Mixed_Mode_States."Start Stabilize" ("MixedModeStates"), s=w1109, f=w1104) -> (s? t:f=w1096:T26)
      }
      frame #10 {
        n500 = local read "Convergence Status"() -> (w1140:T25[])
        n501 = Build Array(MM_Result_Actions."Nop" ("MM Result Actions")) -> (w1137:T1[])
        n502 = local read "Hold Data"() -> (w1134:T8[])
        n503 = local read "Stiffness Limits"() -> (w1136:dbl[][][])
        n504 = for {
          tunnel: T14 {"Displacements"=[], "Forces"=[]} ("Increments") -> [w1167]
          tunnel: [w1156] -> w1141 mode=indexing
          tunnel: w1140 -> [w1160] mode=indexing
          tunnel: w1134 -> [w1158] mode=indexing
          tunnel: w1139 -> [w1157] mode=indexing
          tunnel: w1136 -> [w1155] mode=indexing
          tunnel: [w1152] -> w1131 mode=indexing
          tunnel: [w1151] -> w1130 mode=indexing
          i -> [w1154]
          n505 = Unbundle By Name(w1157) -> ("Displacement \nCommands"=w1165:dbl[], "Forces"=w1163:dbl[])
          n506 = Unbundle By Name(w1158) -> ("Forces"=w1159:dbl[], "Displacement \nCommands"=w1153:dbl[])
          n507 = Subtract(x=w1159, y=w1163) -> (x-y=w1162:dbl[])
          n508 = Subtract(x=w1153, y=w1165) -> (x-y=w1164:dbl[])
          n509 = call "Calculated Stiffness Jacobian.vi"("LBCB Number"=w1154, "Actions"=Persistant_DAO_Actions."Get" ("Stiffness Jacobian Datastore Actions")) -> ("Stiffness Jacobian Out"=w1170:T24)  [unwired: 2 in, 7 out]
          n510 = Bundle By Name(cluster=w1167, "Displacements"=w1164, "Forces"=w1162) -> (w1166:T14)
          n511 = call "Update Stiffness Jacobian.vi"("Stiffness Limit"=w1155, "Mixed Mode Convergence Status In"=w1160, "Increments"=w1166, "Stiffness Jacobian In"=w1170) -> ("Jacobian Stiffness Column"=w1152:T3, "Stiffness Jacobian Out"=w1169:T24, "Updated"=w1151:bool)  [unwired: 5 out]
          n512 = call "Calculated Stiffness Jacobian.vi"("Stiffness Jacobian In"=w1169, "LBCB Number"=w1154, "Actions"=Persistant_DAO_Actions."Set" ("Stiffness Jacobian Datastore Actions")) -> ("Stiffness Jacobian Out"=w1161:T24)  [unwired: 1 in, 7 out]
          n513 = Bundle("Stiffness Jacobian Out"=w1161) -> (w1156:cluster{"Stiffness Jacobian Out":T24})  [unwired: 1 in]
        }
        n514 = Or Array Elements(Boolean array=w1130) -> (logical OR=w1129:bool)
        n515 = case shown="True" w1129 {
          tunnel: w1128 -> [w1147 w1150]
          tunnel: [w1147 w1148] -> w1127
          frame #0 {
          }
          frame #1 {
            n516 = Enqueue Element(queue=w1150, element=Command_or_Stiffness_Updates."Stiffness Update") -> (queue out=w1148:refnum<queue>)  [unwired: 2 in, 2 out]
          }
        }
        n517 = local write "Stiffness Jacobian Column"(w1131) -> ()
        n518 = local write "Stiffness Jacobian"(w1141) -> ()
      }
      frame #11 {
        w1186 = DAO_Actions."Get" ("Mixed Mode Commands\n Datastore Actions")
        n519 = local read "Hold Data"() -> (w1176:T8[])
        n520 = call "Mixed Mode Commands DAO.vi"("Mixed Mode Commands\n Datastore Actions"=w1186) -> ("Current Target"=w1189:T5[])  [unwired: 3 in, 7 out]
        n521 = Build Array(MM_Result_Actions."Nop" ("MM Result Actions")) -> (w1178:T1[])
        n522 = local read "Max Increment"() -> (w1180:dbl[][])
        n523 = local read "Jacobian Gain"() -> (w1181:dbl[][])
        n524 = for {
          tunnel: w1189 -> [w1194] mode=indexing
          tunnel: w1186 -> [w1205]
          tunnel: [w1202] -> w1185 mode=indexing
          tunnel: w1182 -> [w1197] mode=indexing
          tunnel: w1181 -> [w1201] mode=indexing
          tunnel: w1180 -> [w1200] mode=indexing
          tunnel: w1176 -> [w1199] mode=indexing
          tunnel: w1173 -> [w1193] mode=indexing
          n525 = Unbundle By Name(w1199) -> ("Forces"=w1192:dbl[])
          n526 = call "Calculated Stiffness Jacobian.vi"("LBCB Number"=w1197, "Actions"=Persistant_DAO_Actions."Get") -> ("Stiffness Jacobian Out"=w1195:T24)  [unwired: 8 in, 1 out]
          n527 = call "Convergence Status DAO.vi"("LBCB Selected"=w1197, "Actions"=w1205) -> ("Convergence Status Out"=w1198:T25)  [unwired: 2 in, 7 out]
          n528 = Unbundle By Name(w1198) -> ("IsConverged"=w1204:bool[])
          n529 = And Array Elements(Boolean array=w1204) -> (logical AND=w1203:bool)
          n530 = case shown="False" w1203 {
            tunnel: [w1210 w1214] -> w1202
            tunnel: w1194 -> [w1211 w1215]
            tunnel: w1192 -> [w1206 _]
            tunnel: w1201 -> [w1208 _]
            tunnel: w1200 -> [w1209 _]
            tunnel: w1198 -> [w1212 _]
            tunnel: w1195 -> [w1207 _]
            tunnel: w1193 -> [_ w1213]
            frame #0 {
              n531 = call "Update Iterative Command.vi"("Stiffness Jacobian In"=w1207, "Maximum Displacement\nIncrement"=w1209, "Jacobian Gain"=w1208, "Convergence Status In"=w1212, "Current Forces"=w1206, "Target  Command Data In"=w1211) -> ("Updated  Command Data Out"=w1210:T5)  [unwired: 5 in]
            }
            frame #1 {
              n532 = call "Command Data 2 Control Target.vi"("Current Command"=w1213, "Current Target"=w1215) -> ("Output"=w1214:T5)  [unwired: 1 in, 8 out]
            }
          }
        }
        n533 = call "Mixed Mode Commands DAO.vi"("Current Target In"=w1185, "Mixed Mode Commands\n Datastore Actions"=DAO_Actions."Set" ("Mixed Mode Commands\n Datastore Actions")) -> ("Current Target"=w1184:T5[])  [unwired: 3 in, 6 out]
        n534 = local write "Iterative Target"(w1184) -> ()
      }
      frame #12 {
        w1222 = T1[] [enum."Check Limits", enum."Store Prev Reading", enum."Hold Off", enum."Averaging Off"] items=["Nop", "Set Command", "Check Limits", "Send Command", "Store Prev Reading", "Averaging On", "Averaging Off", "Hold On", "Hold Off", "PID Hold On", "PID Hold Off", "Clear Increment Faults", "Set Initial Position"]
        n535 = Unbundle By Name(w1223) -> ("Ramp Times.Iterative"=w1231:T38)
        n536 = Unbundle By Name(w1231) -> ("Ramp"=w1227:dbl)
        n537 = Equal To 0?(x=w1227) -> (x = 0?=w1228:bool)
        n538 = Select(t=0.1, s=w1228, f=w1227) -> (s? t:f=w1226:dbl)
        n539 = Enqueue Element(queue=w1217, element=Command_or_Stiffness_Updates."Command Update") -> (queue out=w1216:refnum<queue>)  [unwired: 2 in, 2 out]
        n540 = Bundle By Name(cluster=w1231, "Ramp"=w1226) -> (w1229:T38)
      }
      frame #13 {
        w1239 = T1[] [enum."Set Command", enum."Check Limits", enum."Send Command"] items=["Nop", "Set Command", "Check Limits", "Send Command", "Store Prev Reading", "Averaging On", "Averaging Off", "Hold On", "Hold Off", "PID Hold On", "PID Hold Off", "Clear Increment Faults", "Set Initial Position"]
        n541 = call "Ramp Time Completions.vi"("Current Ramp Time"=w1253, "Initial"=w1251) -> ("Still in Ramp"=w1254:bool, "Fraction\nCompleted"=w1255:dbl)
        n542 = case shown="True" w1254 {
          tunnel: w1255 -> [_ w1262]
          tunnel: [Mixed_Mode_States."Start Iterative Stabilize" ("MixedModeStates") Mixed_Mode_States."Run Iterative Ramp" ("MixedModeStates")] -> w1238
          tunnel: [w1257 w1260] -> w1233
          frame #0 {
            n543 = call "Mixed Mode Commands DAO.vi"("Mixed Mode Commands\n Datastore Actions"=DAO_Actions."Get" ("Mixed Mode Commands\n Datastore Actions")) -> ("Current Target"=w1257:T5[])  [unwired: 3 in, 7 out]
          }
          frame #1 {
            n544 = call "Calculate Ramp Displacements.vi"("Iterative\nRamp"=TRUE ("Iterative\nRamp"), "Ramp Time"=w1262) -> ("Target"=w1260:T5[])  [unwired: 1 in]
          }
        }
        n545 = Dequeue Element(queue=w1248, timeout in ms (-1)=w1243) -> (queue out=w1247:refnum<queue>, element=w1249:T41, timed out?=w1250:bool)  [unwired: 1 in, 1 out]
        n546 = Select(t=w1246, s=w1250, f=w1249) -> (s? t:f=w1245:T41)
        n547 = local write "Target"(w1233) -> ()
        n548 = call "MM Command to Cntrl Loop Actuator In.vi"("Target"=w1233, "Current Cartesian Position"=w1234, "Number of\nLBCBs In"=w1244, "LBCB Type"=w1242, "Position"=w1241, "Rigid Connection"=w1237) -> ("Cmd Out"=w1240:T2[])  [unwired: 5 in, 4 out]
      }
      frame #14 {
        w1267 = T1[] [enum."Averaging On", enum."Check Limits"] items=["Nop", "Set Command", "Check Limits", "Send Command", "Store Prev Reading", "Averaging On", "Averaging Off", "Hold On", "Hold Off", "PID Hold On", "PID Hold Off", "Clear Increment Faults", "Set Initial Position"]
        n549 = Unbundle By Name(w1268) -> ("Ramp Times.Iterative"=w1270:T38)
      }
      frame #15 {
        w1276 = T1[] [enum."Averaging On", enum."Check Limits"] items=["Nop", "Set Command", "Check Limits", "Send Command", "Store Prev Reading", "Averaging On", "Averaging Off", "Hold On", "Hold Off", "PID Hold On", "PID Hold Off", "Clear Increment Faults", "Set Initial Position"]
        n550 = Unbundle By Name(w1284) -> ("Stab"=w1289:dbl)
        n551 = Divide(x=w1286, y=u64 1000) -> (x/y=w1288:dbl)
        n552 = Greater?(x=w1288, y=w1289) -> (0:w1285:bool)
        n553 = Dequeue Element(queue=w1281, timeout in ms (-1)=w1277) -> (queue out=w1280:refnum<queue>, element=w1282:T41, timed out?=w1283:bool)  [unwired: 1 in, 1 out]
        n554 = Select(t=w1279, s=w1283, f=w1282) -> (s? t:f=w1278:T41)
        n555 = Select(t=Mixed_Mode_States."Start Iterative Holding" ("MixedModeStates"), s=w1285, f=Mixed_Mode_States."Iterative Stabilize" ("MixedModeStates")) -> (s? t:f=w1275:T26)
      }
      frame #16 {
        w1297 = T1[] [enum."Averaging On", enum."Hold On", enum."Check Limits"] items=["Nop", "Set Command", "Check Limits", "Send Command", "Store Prev Reading", "Averaging On", "Averaging Off", "Hold On", "Hold Off", "PID Hold On", "PID Hold Off", "Clear Increment Faults", "Set Initial Position"]
      }
      frame #17 {
        w1306 = T1[] [enum."Averaging On", enum."Hold On", enum."Check Limits"] items=["Nop", "Set Command", "Check Limits", "Send Command", "Store Prev Reading", "Averaging On", "Averaging Off", "Hold On", "Hold Off", "PID Hold On", "PID Hold Off", "Clear Increment Faults", "Set Initial Position"]
        n556 = Divide(x=w1316, y=u64 1000) -> (x/y=w1318:dbl)
        n557 = Unbundle By Name(w1319) -> ("Hold"=w1315:dbl)
        n558 = Greater?(x=w1318, y=w1315) -> (0:w1314:bool)
        n559 = Dequeue Element(queue=w1311, timeout in ms (-1)=w1307) -> (queue out=w1310:refnum<queue>, element=w1312:T41, timed out?=w1313:bool)  [unwired: 1 in, 1 out]
        n560 = Select(t=w1309, s=w1313, f=w1312) -> (s? t:f=w1308:T41)
        n561 = Select(t=Mixed_Mode_States."Convergence Check" ("MixedModeStates"), s=w1314, f=Mixed_Mode_States."Iterative Holding") -> (s? t:f=w1305:T26)
      }
      frame #18 {
        w1327 = T1[] [enum."Averaging On", enum."Check Limits", enum."PID Hold On"] items=["Nop", "Set Command", "Check Limits", "Send Command", "Store Prev Reading", "Averaging On", "Averaging Off", "Hold On", "Hold Off", "PID Hold On", "PID Hold Off", "Clear Increment Faults", "Set Initial Position"]
        n562 = Unbundle By Name(w1328) -> ("Ramp Times.Initial"=w1330:T38)
      }
      frame #19 {
        w1336 = T1[] [enum."Averaging On", enum."Check Limits", enum."PID Hold On"] items=["Nop", "Set Command", "Check Limits", "Send Command", "Store Prev Reading", "Averaging On", "Averaging Off", "Hold On", "Hold Off", "PID Hold On", "PID Hold Off", "Clear Increment Faults", "Set Initial Position"]
        n563 = Unbundle By Name(w1344) -> ("Stab"=w1349:dbl)
        n564 = Divide(x=w1346, y=u64 1000) -> (x/y=w1348:dbl)
        n565 = Dequeue Element(queue=w1341, timeout in ms (-1)=w1337) -> (queue out=w1340:refnum<queue>, element=w1342:T41, timed out?=w1343:bool)  [unwired: 1 in, 1 out]
        n566 = Greater?(x=w1348, y=w1349) -> (0:w1345:bool)
        n567 = Select(t=w1339, s=w1343, f=w1342) -> (s? t:f=w1338:T41)
        n568 = Select(t=Mixed_Mode_States."Start Hold" ("MixedModeStates"), s=w1345, f=Mixed_Mode_States."Stabilize" ("MixedModeStates")) -> (s? t:f=w1335:T26)
      }
      frame #20 {
        w1357 = T1[] [enum."Averaging On", enum."Check Limits", enum."PID Hold On", enum."Hold On"] items=["Nop", "Set Command", "Check Limits", "Send Command", "Store Prev Reading", "Averaging On", "Averaging Off", "Hold On", "Hold Off", "PID Hold On", "PID Hold Off", "Clear Increment Faults", "Set Initial Position"]
      }
      frame #21 {
        w1366 = T1[] [enum."Averaging On", enum."Check Limits", enum."PID Hold On", enum."Hold On"] items=["Nop", "Set Command", "Check Limits", "Send Command", "Store Prev Reading", "Averaging On", "Averaging Off", "Hold On", "Hold Off", "PID Hold On", "PID Hold Off", "Clear Increment Faults", "Set Initial Position"]
        n569 = Unbundle By Name(w1379) -> ("Hold"=w1375:dbl)
        n570 = Divide(x=w1376, y=u64 1000) -> (x/y=w1378:dbl)
        n571 = Greater?(x=w1378, y=w1375) -> (0:w1374:bool)
        n572 = Dequeue Element(queue=w1371, timeout in ms (-1)=w1367) -> (queue out=w1370:refnum<queue>, element=w1372:T41, timed out?=w1373:bool)  [unwired: 1 in, 1 out]
        n573 = Select(t=w1369, s=w1373, f=w1372) -> (s? t:f=w1368:T41)
        n574 = Select(t=Mixed_Mode_States."Done" ("MixedModeStates"), s=w1374, f=Mixed_Mode_States."Holding") -> (s? t:f=w1365:T26)
      }
      frame #22 {
        w1388 = T1[] [enum."Averaging Off", enum."Hold Off", enum."PID Hold Off"] items=["Nop", "Set Command", "Check Limits", "Send Command", "Store Prev Reading", "Averaging On", "Averaging Off", "Hold On", "Hold Off", "PID Hold On", "PID Hold Off", "Clear Increment Faults", "Set Initial Position"]
        n575 = Wait Until Next ms Multiple(millisecond multiple=w1386) -> ()  [unwired: 1 out]
      }
      frame #23 {
        w1396 = T1[] [enum."Averaging Off", enum."Hold Off", enum."PID Hold Off"] items=["Nop", "Set Command", "Check Limits", "Send Command", "Store Prev Reading", "Averaging On", "Averaging Off", "Hold On", "Hold Off", "PID Hold On", "PID Hold Off", "Clear Increment Faults", "Set Initial Position"]
      }
      frame #24 {
        n576 = Build Array(MM_Result_Actions."Nop" ("MM Result Actions")) -> (w1405:T1[])
      }
    }
    n577 = for {
      tunnel: w557 -> [w635] mode=indexing
      tunnel: w576 -> [w634] mode=indexing
      tunnel: [w633] -> w577 mode=indexing
      n578 = Bundle By Name(cluster=w634, "Act Cmd"=w635) -> (w633:T2)
    }
    n579 = Equal?(x=w585, y=w584) -> (x = y?=w586:bool)
    n580 = Array Size(array=w580) -> (size(s)=w579:i32)
    n581 = case shown="True" w586 {
      tunnel: w590 -> [w800 w805]
      tunnel: [w800 w804] -> w589
      tunnel: w588 -> [w799 w803]
      tunnel: [w799 w802] -> w587
      tunnel: w585 -> [_ w801]
      frame #0 {
      }
      frame #1 {
        n582 = Enqueue Element(queue=w805, element=w801, error in (no error)=w803) -> (queue out=w804:refnum<queue>, error out=w802:errorcluster)  [unwired: 1 in, 1 out]
      }
    }
    n583 = while {
      shift-right: [w662] -> w613
      shift-left: w578 -> [w645]
      shift-right: [w661] -> w612
      shift-left: w577 -> [w660]
      tunnel: w580 -> [w659] mode=indexing
      shift-right: [w658] -> w611
      shift-left: w608 -> [w657]
      tunnel: w610 -> [w656]
      tunnel: w581 -> [w655]
      tunnel: w607 -> [w654]
      shift-right: [w650] -> w595
      shift-left: w606 -> [w653]
      shift-right: [w649] -> w596
      shift-left: w605 -> [w652]
      shift-right: [w648] -> w597
      shift-left: w604 -> [w651]
      shift-right: [w647] -> w593
      shift-left: w594 -> [w646]
      shift-right: [w644] -> w583
      shift-left: w582 -> [w643]
      tunnel: w569 -> [w642]
      tunnel: w579 -> [w638]
      tunnel: w575 -> [w636]
      i -> [w639]
      stop <- w641 stop-if-true
      # "Previous\nReading"
      # "Measurements"
      # "Current \nCommands"
      # "Previous\nCommands"
      # "Limits Check"
      n584 = local write "MM Result Actions"(w659) -> ()
      n585 = case shown="\"Check Limits\"" w659 {
        tunnel: [w664 w683 w689 w697 w705 w713 w721 w729 w746 w760 w774 w783 w793] -> w662
        tunnel: [w670 w671 w693 w702 w710 w718 w726 w733 w751 w754 w773 w782 w798] -> w661
        tunnel: w660 -> [w670 w685 w693 w702 w710 w718 w726 w733 w751 w757 w771 w782 w798]
        tunnel: [w669 w684 w694 w703 w711 w719 w727 w734 w752 w761 w775 w784 w791] -> w658
        tunnel: w657 -> [w669 w684 w694 w703 w711 w719 w727 w734 w752 w761 w775 w784 _]
        tunnel: w656 -> [_ _ _ _ _ _ _ _ _ w754 w773 _ _]
        tunnel: w655 -> [_ w682 _ _ _ _ _ _ _ _ _ _ _]
        tunnel: w654 -> [_ w681 _ _ _ _ _ _ _ _ _ _ _]
        tunnel: [w668 w680 TRUE w700 w709 w717 w724 FALSE w750 w764 w778 w787 w797] -> w650
        tunnel: w653 -> [w668 w680 _ w700 w709 w717 w724 _ w750 w764 w778 w787 w797]
        tunnel: [w667 w679 w692 TRUE w708 w716 FALSE w732 w749 w763 w777 w786 w796] -> w649
        tunnel: w652 -> [w667 w679 w692 _ w708 w716 _ w732 w749 w763 w777 w786 w796]
        tunnel: [w666 w678 w691 w699 TRUE FALSE w723 w731 w748 w762 w776 w785 w795] -> w648
        tunnel: w651 -> [w666 w678 w691 w699 _ _ w723 w731 w748 w762 w776 w785 w795]
        tunnel: [w665 w675 w690 w698 w706 w714 w722 w730 w747 w756 w772 w779 w794] -> w647
        tunnel: w646 -> [w665 w674 w690 w698 w706 w714 w722 w730 w747 w758 w772 w780 w794]
        tunnel: w645 -> [w664 _ w689 w697 w705 w713 w721 w729 w746 w760 w774 w783 w793]
        tunnel: [w663 w677 w688 w696 w704 w712 w720 w728 w745 w753 w771 w781 w792] -> w644
        tunnel: w643 -> [w663 w677 w688 w696 w704 w712 w720 w728 w745 w753 _ w781 w792]
        tunnel: w642 -> [_ w672 _ _ _ _ _ _ _ _ _ _ _]
        tunnel: [_ w676 _ _ _ _ _ _ _ _ _ _ _] -> w640
        tunnel: w636 -> [_ _ _ _ _ _ _ _ _ w755 _ _ _]
        frame #0 {
        }
        frame #1 {
          # "For Rigid Connection Forces and Displacements\nare checked with individual LBCB readings then \ncombined"
          # "We set commands\nhere even during an abort because\nwe want to show what the exceeded \nlimits are"
          # "Collect Measurements and Check Limits"
          n586 = local read "Actuator Meas. Disp & Forces"() -> (w687:dbl[][])
          n587 = local read "Limits"() -> (w686:T20[])
          n588 = call "Collect All Measurements.vi"("Rigid Connection"=w672, "Limits"=w686, "Position"=w681, "Type"=w682, "Actuator Meas. Disp & Forces"=w687, "Cmd In"=w685, "Within Limits In"=w674) -> ("Within Limits Out"=w675:T16[], "Cart Meas. Disp & Forces"=w673:dbl[][], "Measurements Out"=w683:T23[], "Cmds Out"=w671:T2[])  [unwired: 1 in]
          n589 = local write "Cart Meas. Disp & Forces"(w673) -> ()
          n590 = call "Check For Abort.vi"("Within Limits"=w675) -> ("Faulted"=w676:bool)  [unwired: 1 in, 1 out]
          n591 = local write "Commands"(w671) -> ()
          n592 = local write "Limits Check"(w675) -> ()
          n593 = local write "Measurements"(w683) -> ()
        }
        frame #2 {
        }
        frame #3 {
        }
        frame #4 {
        }
        frame #5 {
        }
        frame #6 {
        }
        frame #7 {
        }
        frame #8 {
          n594 = Index Array(array=w751, index #1=0 ("index"), index #2=1 ("index")) -> (element #1=w743:T2, element #2=w740:T2)
          n595 = Unbundle By Name(w743) -> ("Act Cmd"=w744:dbl[], "Cart Cmd"=w737:dbl[])
          n596 = Unbundle By Name(w740) -> ("Act Cmd"=w739:dbl[], "Cart Cmd"=w736:dbl[])
          n597 = local write "L1 Ctrl Loop In Actuator"(w744) -> ()
          n598 = local write "L2 Ctrl Loop In Actuator"(w739) -> ()
          n599 = call "Current Position DAO.vi"("LBCB 2 Commands In"=w736, "LBCB 1 Commands In"=w737, "Actions"=DAO_Actions."Set") -> ()  [unwired: 7 in, 2 out]
        }
        frame #9 {
          # "\"Set Command\" is supposed to be followed by\n\"Check Limits\".  At that point an increment fault\nwill abort the command"
          n600 = local read "Increment Limits"() -> (w759:T2[])
          n601 = for {
            tunnel: w759 -> [w770] mode=indexing
            tunnel: w758 -> [w769] mode=indexing
            tunnel: w754 -> [w765] mode=indexing
            tunnel: w757 -> [w768] mode=indexing
            tunnel: [w767] -> w756 mode=indexing
            tunnel: w755 -> [w766] mode=indexing
            n602 = call "Calculate Increment.vi"("LBCB Number"=w766, "Increment Limits"=w770, "Previous"=w768, "Current"=w765, "Within Limits In"=w769) -> ("Within Limits Out"=w767:T16)  [unwired: 5 in, 1 out]
          }
        }
        frame #10 {
        }
        frame #11 {
          n603 = for {
            tunnel: w780 -> [w790] mode=indexing
            tunnel: [w789] -> w779 mode=indexing
            w788 = TRUE ("Increments.Dx")
            n604 = Bundle By Name(cluster=w790, "Act Incr.X1"=w788, "Act Incr.X2"=w788, "Act Incr.Y1"=w788, "Act Incr.Z1"=w788, "Act Incr.Z2"=w788, "Act Incr.Z3"=w788, "Cart Incr.Dx"=w788, "Cart Incr.Dy"=w788, "Cart Incr.Dz"=w788, "Cart Incr.Rx"=w788, "Cart Incr.Ry"=w788, "Cart Incr.Rz"=w788) -> (w789:T16)
          }
        }
        frame #12 {
          # "Store for Stiffness\nJacobian Previous Target"
          n605 = local read "Hold Data"() -> (w791:T8[])
        }
      }
      n606 = Greater Or Equal?(x=w639, y=w638) -> (x >= y?=w637:bool)
      n607 = Or(x=w640, y=w637) -> (x .or. y?=w641:bool)
    }
    "Collecting DAQ Samples" <- w595
    n608 = call "GetSamplingRate.vi"() -> ("Sampling"=w616:i32)
    n609 = local write "Mixed Mode"(w616) -> ()
    n610 = local read "PID Control"() -> (w598:T27[])
    n611 = case shown="\"Start Initial Ramp\", Default" w585 {
      tunnel: w593 -> [_ _ _ _ _ _ _ w815 _]
      tunnel: [w806 w807 w808 w809 w810 w811 w812 w814 w816] -> w592
      tunnel: w591 -> [w806 w807 w808 w809 w810 w811 w812 w813 w816]
      frame #0 {
      }
      frame #1 {
      }
      frame #2 {
      }
      frame #3 {
      }
      frame #4 {
      }
      frame #5 {
      }
      frame #6 {
      }
      frame #7 {
        n612 = call "Check For Abort.vi"("Mixed Mode State In"=w813, "Within Limits"=w815) -> ("Mixed Mode State Out"=w814:T26)  [unwired: 1 out]
      }
      frame #8 {
      }
    }
    n613 = for {
      tunnel: [w819] -> w599 mode=indexing
      tunnel: w598 -> [w818] mode=indexing
      tunnel: w597 -> [w817]
      n614 = Unbundle By Name(w818) -> ("I-Control"=w821:bool, "Ctrl Mode"=w820:bool)
      n615 = Compound Arithmetic op=AND(w821, w820, w817) -> (w819:bool)
    }
    n616 = Not Equal?(x=w592, y=w585) -> (x != y?=w625:bool)
    n617 = local write "Averaging"(w595) -> ()
    n618 = case shown="True" w625 {
      tunnel: w589 -> [w1413 w1418]
      tunnel: [w1413 w1417] -> w626
      tunnel: w587 -> [w1412 w1416]
      tunnel: [w1412 w1415] -> w621
      tunnel: w592 -> [_ w1414]
      frame #0 {
      }
      frame #1 {
        n619 = Enqueue Element(queue=w1418, element=w1414, error in (no error)=w1416) -> (queue out=w1417:refnum<queue>, error out=w1415:errorcluster)  [unwired: 1 in, 1 out]
      }
    }
    n620 = local read "App Running"() -> (w617:bool)
    n621 = Index Array(array=w599, index #1=0 ("index"), index #2=1 ("index")) -> (element #1=w602:bool, element #2=w603:bool)
    n622 = local write "MixedModeStates"(w592) -> ()
    n623 = local write "Hold Period"(w596) -> ()
    n624 = Not(x=w617) -> (.not. x?=w615:bool)
    n625 = local write "L1 PID On"(w602) -> ()
    n626 = local write "L2 PID On"(w603) -> ()
  }
  n627 = call "Autobalance Initial State DAO.vi"() -> ("autobalance\nfile"=w103:string, "Initial Values"=w107:T10[])  [unwired: 3 in, 7 out]
  n628 = Initialize Array(0.0 ("element"), 6 ("dimension size")) -> (w54:dbl[])
  n629 = call "Autobalance Initial State DAO.vi"() -> ("Initial Values"=w102:T10[])  [unwired: 3 in, 8 out]
  n630 = while {
    shift-right: [w1438] -> _
    shift-left: w54 -> [w1441]
    tunnel: w80 -> [w1440]
    shift-right: [w1433] -> _
    shift-left: w107 -> [w1436]
    tunnel: LBCB_Number."LBCB1" ("LBCB Number") -> [w1435]
    tunnel: [w1434] -> w99
    shift-right: [w1432] -> _
    shift-left: Autobalance_State."Init" ("Autobalance State Out") -> [w1431]
    shift-right: [w1430] -> _
    shift-left: _ -> [w1429]
    shift-right: [w1428] -> _
    shift-left: _ -> [w1427]
    tunnel: w68 -> [w1426]
    stop <- w1434 stop-if-true
    # "LBCB 1 Control Loop"
    # "Cartesian\nCommand\nNo  Offset"
    # "Actuator Command"
    n631 = local read "L1 Ctrl Loop In Actuator"() -> (w1425:dbl[])
    n632 = call "GetSamplingRate.vi"() -> ("Sampling"=w1439:i32)
    n633 = local read "App Running"() -> (w1442:bool)
    n634 = local read "L1 Ctrl Loop State"() -> (w1443:T15)
    n635 = local write "L1 Control Rate"(w1439) -> ()
    n636 = Not(x=w1442) -> (.not. x?=w1434:bool)
    n637 = case shown="\"On\"" w1443 {
      tunnel: w1439 -> [_ _ _ _ _ _ w1526]
      tunnel: [w1448 w1454 w1462 w1464 w1499 w1509 w1518] -> w1438
      tunnel: w1441 -> [w1448 w1454 w1462 _ _ w1509 _]
      tunnel: w1440 -> [w1449 w1455 w1463 w1475 w1498 w1510 w1525]
      tunnel: w1435 -> [_ _ _ w1469 w1497 _ w1524]
      tunnel: w1425 -> [_ _ _ _ _ _ w1512]
      tunnel: [w1447 w1453 w1461 w1473 w1492 w1508 w1521] -> w1428
      tunnel: [w1450 w1456 w1459 w1465 w1489 w1511 w1517] -> w1433
      tunnel: w1436 -> [w1450 w1456 _ w1466 w1490 w1511 w1517]
      tunnel: [w1446 w1452 Autobalance_State."Init" ("Autobalance State Out") w1468 w1495 w1507 w1516] -> w1432
      tunnel: w1431 -> [w1446 w1452 _ w1468 w1496 w1507 w1516]
      tunnel: [w1445 w1451 T11 TRUE ("InitialPosition? Out") w1467 w1493 w1506 w1515] -> w1430
      tunnel: w1429 -> [w1445 w1451 _ w1467 w1494 w1506 w1515]
      tunnel: w1427 -> [_ _ _ _ w1491 _ _]
      tunnel: w1426 -> [_ _ _ _ w1485 _ _]
      frame #0 {
        n638 = Wait Until Next ms Multiple(millisecond multiple=u32 1000) -> ()  [unwired: 1 out]
        n639 = Divide(x=w1448, y=w1449) -> (x/y=w1447:dbl[])
      }
      frame #1 {
        n640 = Divide(x=w1454, y=w1455) -> (x/y=w1453:dbl[])
      }
      frame #2 {
        n641 = call "Autobalance Initial State DAO.vi"() -> ("Initial Values"=w1459:T10[])  [unwired: 2 in, 9 out]
        n642 = local write "L1 Ctrl Loop State"(Control_Loop_State."Autobalancing" ("L1 Ctrl Loop State")) -> ()
        n643 = Divide(x=w1462, y=w1463) -> (x/y=w1461:dbl[])
      }
      frame #3 {
        n644 = call "Initial Command DAO.vi"("LBCB Number"=w1469, "DAO Actions"=DAO_Actions."Get") -> ("Command Out"=w1471:T46)  [unwired: 2 in, 7 out]
        n645 = call "Actuator Point 2 Array.vi"("Actuator Point"=w1471) -> ("Array"=w1464:dbl[])
        n646 = for {
          tunnel: w1466 -> [w1478] mode=indexing
          tunnel: [w1476] -> w1465 mode=indexing
          n647 = Bundle By Name(cluster=w1478, "IsBalanced"=T11 TRUE) -> (w1476:T10)
        }
        n648 = local write "L1 Ctrl Loop In Actuator"(w1464) -> ()
        n649 = local write "L1 Ctrl Loop State"(Control_Loop_State."Ready for Control" ("L1 Ctrl Loop State")) -> ()
        n650 = Divide(x=w1464, y=w1475) -> (x/y=w1473:dbl[])
        n651 = call "Daq Send.vi"("LBCB Select"=w1469, "Commands"=w1473, "Daq Actions"=Daq_Actions."Send Commands") -> ()  [unwired: 2 in, 7 out]
      }
      frame #4 {
        n652 = local read "Auto Balance Error Tolerance"() -> (w1483:dbl[][])
        n653 = local read "Servo Error"() -> (w1486:dbl[][])
        n654 = Index Array(array=w1486, index (row)=0 ("disabled index (col)")) -> (element=w1484:dbl[])  [unwired: 1 in]
        n655 = local read "AB Parameters"() -> (w1479:T7)
        n656 = Subtract(x=w1484, y=w1485) -> (x-y=w1487:dbl[])
        n657 = Index Array(array=w1483, index (row)=0 ("disabled index (col)")) -> (element=w1482:dbl[])  [unwired: 1 in]
        n658 = call "Autobalance.vi"("Servo Errors"=w1487, 1:"Autobalance State In"=w1496, "LBCB Number"=w1497, "InitialPosition? In"=w1494, "Error Tolerance"=w1482, "Command In"=w1491, 11:"Autobalance State In"=w1490, "Autobalance \nControl Parameters"=w1479) -> ("IsBalanced"=w1488:T11, "Command Out"=w1492:dbl[], "InitialPosition? Out"=w1493:T11, 14:"Autobalance State Out"=w1495:T37, 15:"Autobalance State Out"=w1489:T10[])  [unwired: 3 out]
        n659 = Multiply(x=w1498, y=w1492) -> (x*y=w1499:dbl[])
        n660 = case shown="True" w1488 {
          tunnel: w1499 -> [_ w1504]
          tunnel: w1497 -> [_ w1502]
          frame #0 {
          }
          frame #1 {
            n661 = call "Array 2 Actuator Point.vi"("Array"=w1504) -> ("Actuator Point"=w1505:T46)
            n662 = call "Initial Command DAO.vi"("Command In"=w1505, "LBCB Number"=w1502, "DAO Actions"=DAO_Actions."Set") -> ()  [unwired: 1 in, 8 out]
            n663 = local write "L1 Ctrl Loop State"(Control_Loop_State."Set Command" ("L1 Ctrl Loop State")) -> ()
          }
        }
        n664 = call "Daq Send.vi"("LBCB Select"=w1497, "Commands"=w1492, "Daq Actions"=Daq_Actions."Send Commands") -> ()  [unwired: 2 in, 7 out]
      }
      frame #5 {
        n665 = Divide(x=w1509, y=w1510) -> (x/y=w1508:dbl[])
      }
      frame #6 {
        w1513 = 0 ("disabled index (col)")
        # "4. Actiator and Cartesian Limit Check"
        # "3. Actuator to Cartesian, Cartesian to Actuator Conversions"
        n666 = local read "Actuator Meas. Disp & Forces"() -> (w1523:dbl[][])
        n667 = Divide(x=w1526, y=1000.0) -> (x/y=w1528:dbl)
        n668 = local read "L1 PID On"() -> (w1522:bool)
        n669 = Index Array(array=w1523, index (row)=w1513) -> (element=w1514:dbl[])  [unwired: 1 in]
        n670 = Delete From Array(array=w1514, length=6, index=w1513) -> (array with subset deleted=w1520:dbl[])  [unwired: 1 out]
        n671 = case shown="False" w1522 {
          tunnel: [w1530 w1536] -> w1518
          tunnel: w1520 -> [_ w1535]
          tunnel: w1512 -> [w1532 w1533]
          tunnel: w1528 -> [_ w1534]
          frame #0 {
            n672 = local read "L1 I Const"() -> (w1531:dbl[])
            n673 = Add(x=w1532, y=w1531) -> (x+y=w1530:dbl[])
          }
          frame #1 {
            n674 = Subtract(x=w1533, y=w1535) -> (x-y=w1541:dbl[])
            n675 = local read "L1 I Gain"() -> (w1542:dbl[])
            n676 = local read "L1 P Gain"() -> (w1537:dbl[])
            n677 = local read "L1 I Const"() -> (w1538:dbl[])
            n678 = Multiply(x=w1541, y=w1537) -> (x*y=w1539:dbl[])
            n679 = Compound Arithmetic op=MULTIPLY(w1541, w1542, w1534) -> (w1543:dbl[])
            n680 = Add(x=w1543, y=w1538) -> (x+y=w1540:dbl[])
            n681 = Compound Arithmetic op=ADD(w1533, w1539, w1540) -> (w1536:dbl[])
            n682 = local write "L1 I Const"(w1540) -> ()
          }
        }
        n683 = Divide(x=w1518, y=w1525) -> (x/y=w1521:dbl[])
        n684 = call "Daq Send.vi"("LBCB Select"=w1524, "Commands"=w1521, "Daq Actions"=Daq_Actions."Send Commands") -> ()  [unwired: 2 in, 7 out]
      }
    }
    n685 = local write "L1 Ctrl Loop Out Actuator"(w1438) -> ()
    n686 = local write "L1 Autobalance Out"(w1433) -> ()
    n687 = local write "L1 Cmd  Volts"(w1428) -> ()
    n688 = Wait Until Next ms Multiple(millisecond multiple=u32 6) -> ()  [unwired: 1 out]
  }
  n689 = while {
    tunnel: [w1553] -> _
    shift-right: [w1558] -> _
    shift-left: _ -> [w1560]
    tunnel: w75 -> [w1559]
    shift-right: [w1552] -> _
    shift-left: w102 -> [w1557]
    tunnel: LBCB_Number."LBCB2" ("LBCB Number") -> [w1555]
    tunnel: [w1553] -> w98
    shift-right: [w1551] -> _
    shift-left: _ -> [w1550]
    shift-right: [w1549] -> _
    shift-left: _ -> [w1547]
    shift-right: [w1548] -> _
    shift-left: _ -> [w1546]
    tunnel: w9 -> [_]
    tunnel: w67 -> [w1545]
    stop <- w1553 stop-if-true
    # "LBCB 2 Control Loop"
    # "Cartesian\nCommand\nNo  Offset"
    # "Actuator Command"
    n690 = local read "L2 Ctrl Loop In Actuator"() -> (w1544:dbl[])
    n691 = call "GetSamplingRate.vi"() -> ("Sampling"=w1554:i32)
    n692 = local read "App Running"() -> (w1561:bool)
    n693 = local read "L2 Ctrl Loop State"() -> (w1562:T15)
    n694 = local write "L2 Control Rate"(w1554) -> ()
    n695 = Not(x=w1561) -> (.not. x?=w1553:bool)
    n696 = case shown="\"On\"" w1562 {
      tunnel: w1554 -> [_ _ _ _ _ _ w1647]
      tunnel: [w1566 w1576 w1583 w1599 w1611 w1629 w1639] -> w1558
      tunnel: w1560 -> [_ w1576 w1583 _ _ w1629 _]
      tunnel: w1559 -> [w1567 w1575 w1584 w1603 w1618 w1630 w1646]
      tunnel: w1555 -> [_ _ _ w1594 w1617 _ w1645]
      tunnel: w1544 -> [w1566 _ _ _ _ _ w1633]
      tunnel: [w1568 w1574 w1582 w1600 w1619 w1631 w1642] -> w1551
      tunnel: [w1569 w1577 w1581 w1602 w1612 w1628 w1638] -> w1552
      tunnel: w1557 -> [w1569 w1577 _ w1604 w1613 w1628 w1638]
      tunnel: w1550 -> [_ _ _ w1598 _ _ _]
      tunnel: [w1565 w1573 T11 TRUE ("InitialPosition? Out") w1597 w1615 w1627 w1637] -> w1549
      tunnel: [w1564 w1572 Autobalance_State."Init" ("Autobalance State Out") w1596 w1614 w1626 w1636] -> w1548
      tunnel: w1547 -> [w1565 w1573 _ w1595 w1615 w1627 w1637]
      tunnel: w1546 -> [w1564 w1572 _ w1593 w1614 w1626 w1636]
      tunnel: w1545 -> [_ _ _ w1591 _ _ _]
      frame #0 {
        n697 = Wait Until Next ms Multiple(millisecond multiple=500) -> ()  [unwired: 1 out]
        n698 = Wait Until Next ms Multiple(millisecond multiple=u32 1000) -> ()  [unwired: 1 out]
        n699 = Wait Until Next ms Multiple(millisecond multiple=u32 500) -> ()  [unwired: 1 out]
        n700 = Divide(x=w1566, y=w1567) -> (x/y=w1568:dbl[])
      }
      frame #1 {
        n701 = Divide(x=w1576, y=w1575) -> (x/y=w1574:dbl[])
      }
      frame #2 {
        n702 = local write "L2 Ctrl Loop State"(Control_Loop_State."Autobalancing" ("L1 Ctrl Loop State")) -> ()
        n703 = call "Autobalance Initial State DAO.vi"() -> ("Initial Values"=w1581:T10[])  [unwired: 2 in, 9 out]
        n704 = Divide(x=w1583, y=w1584) -> (x/y=w1582:dbl[])
      }
      frame #3 {
        w1586 = 1 ("disabled index (col)")
        n705 = local read "Auto Balance Error Tolerance"() -> (w1590:dbl[][])
        n706 = local read "Servo Error"() -> (w1588:dbl[][])
        n707 = local read "AB Parameters"() -> (w1585:T7)
        n708 = Index Array(array=w1588, index (row)=w1586) -> (element=w1587:dbl[])  [unwired: 1 in]
        n709 = Index Array(array=w1590, index (row)=w1586) -> (element=w1589:dbl[])  [unwired: 1 in]
        n710 = Subtract(x=w1587, y=w1591) -> (x-y=w1592:dbl[])
        n711 = call "Autobalance.vi"("Servo Errors"=w1592, 1:"Autobalance State In"=w1593, "LBCB Number"=w1594, "InitialPosition? In"=w1595, "Error Tolerance"=w1589, "Command In"=w1598, 11:"Autobalance State In"=w1604, "Autobalance \nControl Parameters"=w1585) -> ("IsBalanced"=w1601:T11, "Command Out"=w1600:dbl[], "InitialPosition? Out"=w1597:T11, 14:"Autobalance State Out"=w1596:T37, 15:"Autobalance State Out"=w1602:T10[])  [unwired: 3 out]
        n712 = Multiply(x=w1600, y=w1603) -> (x*y=w1599:dbl[])
        n713 = case shown="True" w1601 {
          tunnel: w1594 -> [_ w1608]
          tunnel: w1599 -> [_ w1607]
          frame #0 {
          }
          frame #1 {
            n714 = call "Array 2 Actuator Point.vi"("Array"=w1607) -> ("Actuator Point"=w1609:T46)
            n715 = local write "L2 Ctrl Loop State"(Control_Loop_State."Set Command" ("L1 Ctrl Loop State")) -> ()
            n716 = call "Initial Command DAO.vi"("Command In"=w1609, "LBCB Number"=w1608, "DAO Actions"=DAO_Actions."Set") -> ()  [unwired: 1 in, 8 out]
          }
        }
        n717 = call "Daq Send.vi"("LBCB Select"=w1594, "Commands"=w1600, "Daq Actions"=Daq_Actions."Send Commands") -> ()  [unwired: 2 in, 7 out]
      }
      frame #4 {
        n718 = call "Initial Command DAO.vi"("LBCB Number"=w1617, "DAO Actions"=DAO_Actions."Get") -> ("Command Out"=w1621:T46)  [unwired: 2 in, 7 out]
        n719 = for {
          tunnel: w1613 -> [w1625] mode=indexing
          tunnel: [w1623] -> w1612 mode=indexing
          n720 = Bundle By Name(cluster=w1625, "IsBalanced"=T11 TRUE) -> (w1623:T10)
        }
        n721 = call "Actuator Point 2 Array.vi"("Actuator Point"=w1621) -> ("Array"=w1611:dbl[])
        n722 = local write "L2 Ctrl Loop In Actuator"(w1611) -> ()
        n723 = local write "L2 Ctrl Loop State"(Control_Loop_State."Ready for Control" ("L1 Ctrl Loop State")) -> ()
        n724 = Divide(x=w1611, y=w1618) -> (x/y=w1619:dbl[])
        n725 = call "Daq Send.vi"("LBCB Select"=w1617, "Commands"=w1619, "Daq Actions"=Daq_Actions."Send Commands") -> ()  [unwired: 2 in, 7 out]
      }
      frame #5 {
        n726 = Divide(x=w1629, y=w1630) -> (x/y=w1631:dbl[])
      }
      frame #6 {
        # "4. Actiator and Cartesian Limit Check"
        # "3. Actuator to Cartesian, Cartesian to Actuator Conversions"
        n727 = local read "Actuator Meas. Disp & Forces"() -> (w1644:dbl[][])
        n728 = Divide(x=w1647, y=1000.0) -> (x/y=w1649:dbl)
        n729 = local read "L2 PID On"() -> (w1643:bool)
        n730 = Index Array(array=w1644, index (row)=1) -> (element=w1635:dbl[])  [unwired: 1 in]
        n731 = Delete From Array(array=w1635, length=6, index=0) -> (array with subset deleted=w1641:dbl[])  [unwired: 1 out]
        n732 = case shown="False" w1643 {
          tunnel: [w1651 w1658] -> w1639
          tunnel: w1641 -> [_ w1657]
          tunnel: w1633 -> [w1653 w1655]
          tunnel: w1649 -> [_ w1656]
          frame #0 {
            n733 = local read "L2 I Const"() -> (w1652:dbl[])
            n734 = Add(x=w1653, y=w1652) -> (x+y=w1651:dbl[])
          }
          frame #1 {
            n735 = local read "L2 I Gain"() -> (w1654:dbl[])
            n736 = Subtract(x=w1655, y=w1657) -> (x-y=w1663:dbl[])
            n737 = local read "L2 P Gain"() -> (w1659:dbl[])
            n738 = local read "L2 I Const"() -> (w1660:dbl[])
            n739 = Multiply(x=w1663, y=w1659) -> (x*y=w1661:dbl[])
            n740 = Compound Arithmetic op=MULTIPLY(w1663, w1654, w1656) -> (w1664:dbl[])
            n741 = Add(x=w1664, y=w1660) -> (x+y=w1662:dbl[])
            n742 = Compound Arithmetic op=ADD(w1655, w1661, w1662) -> (w1658:dbl[])
            n743 = local write "L2 I Const"(w1662) -> ()
          }
        }
        n744 = Divide(x=w1639, y=w1646) -> (x/y=w1642:dbl[])
        n745 = call "Daq Send.vi"("LBCB Select"=w1645, "Commands"=w1642, "Daq Actions"=Daq_Actions."Send Commands") -> ()  [unwired: 2 in, 7 out]
      }
    }
    n746 = local write "L2 Ctrl Loop Out Actuator"(w1558) -> ()
    n747 = local write "L2 Cmd  Volts"(w1551) -> ()
    n748 = local write "L2 Autobalance Out"(w1552) -> ()
    n749 = Wait Until Next ms Multiple(millisecond multiple=u32 6) -> ()  [unwired: 1 out]
  }
  n750 = flat-sequence {
    tunnel: [w1671] -> w80
    tunnel: [w1673] -> w79
    tunnel: [w1672] -> w78
    tunnel: w6 -> [_]
    tunnel: [w1666] -> w68
    frame #0 {
      n751 = global read "Global Cache.vi" "L1 Calibrations"() -> (w1665:T54)
      n752 = Unbundle By Name(w1665) -> ("Command Sensitivity"=w1671:dbl[], "Servo Error Offset"=w1666:dbl[], "LVDT Sensitivity"=w1667:dbl[], "LVDT Offset"=w1670:dbl[], "Load Cell Offsets"=w1669:dbl[], "Load Cell Sensitivity"=w1668:dbl[])
      n753 = Build Array (concatenate)(w1670, w1669) -> (w1673:dbl[])
      n754 = Build Array (concatenate)(w1667, w1668) -> (w1672:dbl[])
    }
  }
  n755 = Initialize Array(0.0 ("element"), 2 ("dimension size"), 6 ("dimension size")) -> (w58:dbl[][])
  n756 = while {
    shift-right: [w1689] -> _
    shift-left: w6 -> [w1694]
    tunnel: w79 -> [w1693]
    tunnel: w78 -> [w1692]
    tunnel: w73 -> [w1688]
    tunnel: w74 -> [w1687]
    tunnel: [w1681] -> w100
    tunnel: w46 -> [w1679]
    shift-right: [w1676] -> _
    shift-left: w63 -> [w1678]
    tunnel: w64 -> [w1677]
    shift-right: [w1675] -> _
    shift-left: FALSE -> [w1674]
    stop <- w1681 stop-if-true
    # "DAQ Loop"
    n757 = local read "DAQ Enabled"() -> (w1691:bool)
    n758 = case shown="True" w1691 {
      tunnel: w1694 -> [w1705 w1729]
      tunnel: [w1705 w1725] -> w1689
      tunnel: w1693 -> [_ w1728]
      tunnel: w1692 -> [_ w1727]
      tunnel: w1688 -> [_ w1724]
      tunnel: w1687 -> [_ w1723]
      tunnel: [w1704 w1721] -> w1685
      tunnel: [w1701 w1720] -> w1684
      tunnel: [w1697 w1719] -> w1683
      tunnel: [_ TRUE] -> w1682
      tunnel: [w1701 w1716] -> w1680
      tunnel: w1679 -> [_ w1714]
      tunnel: w1678 -> [w1699 w1713]
      tunnel: w1677 -> [_ w1712]
      tunnel: [w1699 w1711] -> w1676
      tunnel: [w1700 w1708] -> w1675
      tunnel: w1674 -> [w1700 w1707]
      frame #0 {
        w1698 = 2 ("dimension size")
        w1695 = 0.0 ("element")
        w1696 = 6 ("dimension size")
        n759 = Initialize Array(0.0 ("element"), 12 ("dimension size"), w1698) -> (w1701:dbl[][])
        n760 = Initialize Array(w1695, w1696, w1698) -> (w1704:dbl[][])
        n761 = Initialize Array(w1695, w1696) -> (w1697:dbl[])
        n762 = Wait Until Next ms Multiple(millisecond multiple=u32 500) -> ()  [unwired: 1 out]
      }
      frame #1 {
        n763 = local read "Number of \nExternal \nChannels"() -> (w1726:i32)
        n764 = call "Daq Receive.vi"("Daq Actions"=Daq_Actions."Get Responses", "error in (no error)"=w1729) -> ("Responses"=w1717:dbl[], "error out"=w1710:errorcluster)  [unwired: 1 in, 6 out]
        n765 = case shown="True" w1707 {
          selector: w1707 -> [_ w1740]
          tunnel: w1713 -> [w1736 w1741]
          tunnel: w1712 -> [w1738 _]
          tunnel: [w1735 w1741] -> w1711
          tunnel: w1710 -> [w1734 w1739]
          tunnel: [w1733 w1739] -> w1709
          tunnel: [TRUE w1740] -> w1708
          frame #0 {
            n766 = Bundle By Name(cluster=w1738, "Command"=Mixed_Mode_Command_Action."Start Acquisition") -> (w1737:T41)
            n767 = Enqueue Element(queue=w1736, element=w1737, error in (no error)=w1734) -> (queue out=w1735:refnum<queue>, error out=w1733:errorcluster)  [unwired: 1 in, 1 out]
          }
          frame #1 {
          }
        }
        n768 = local write "DAQ Volts"(w1717) -> ()
        n769 = Unbundle By Name(w1710) -> ("status"=w1722:bool)
        n770 = call "Split DAQ Data.vi"("L1 Absolute Offsets"=w1728, "L1 Measured Sensitivities"=w1727, "Number of LBCBs"=w1714, "Responses"=w1717, "L2 Absolute Offsets"=w1723, "L2 Measured Sensitivities"=w1724, "Number of \nExternal \nChannels"=w1726) -> ("Servo Error"=w1721:dbl[][], "LVDT & LC"=w1720:dbl[][], "External Channels"=w1719:dbl[], "Volts LVDT & LC"=w1716:dbl[][])  [unwired: 1 in, 4 out]
        n771 = Wait Until Next ms Multiple(millisecond multiple=u32 6) -> ()  [unwired: 1 out]
        n772 = call <vilib>:"Clear Errors.vi"("error in (no error)"=w1709) -> ("error out"=w1725:errorcluster)  [unwired: 6 out]
        n773 = local write "DAQ Overflow"(w1722) -> ()
      }
    }
    n774 = local write "DAQ Started"(w1682) -> ()
    n775 = local read "App Running"() -> (w1690:bool)
    n776 = local write "Servo Error"(w1685) -> ()
    n777 = call "GetSamplingRate.vi"() -> ("Sampling"=w1686:i32)
    n778 = local write "Actuator Meas. Disp & Forces"(w1684) -> ()
    n779 = local write "Volts LVDT & LC"(w1680) -> ()
    n780 = local write "External Sensors"(w1683) -> ()
    n781 = local write "DAQ Rate"(w1686) -> ()
    n782 = Not(x=w1690) -> (.not. x?=w1681:bool)
  }
  n783 = while {
    shift-right: [w1742] -> _
    shift-left: w58 -> [w1753]
    shift-right: [w1747] -> _
    shift-left: w9 -> [w1749]
    tunnel: w103 -> [w1746]
    tunnel: [w1745] -> w94
    stop <- w1745 stop-if-true
    # "Store Previous Command"
    n784 = local read "L1 Ctrl Loop In Actuator"() -> (w1744:dbl[])
    n785 = local read "L2 Ctrl Loop In Actuator"() -> (w1743:dbl[])
    n786 = Build Array(w1744, w1743) -> (w1742:dbl[][])
    n787 = Not Equal?(x=w1742, y=w1753) -> (x != y?=w1752:bool[][])
    n788 = Or Array Elements(Boolean array=w1752) -> (logical OR=w1751:bool)
    n789 = case shown="False" w1751 {
      tunnel: w1742 -> [_ w1763]
      tunnel: w1749 -> [w1755 w1759]
      tunnel: [w1755 w1757] -> w1748
      tunnel: w1746 -> [_ w1756]
      frame #0 {
      }
      frame #1 {
        n790 = local read "Logging Directory"() -> (w1766:path)
        n791 = Build Path(base path=w1766, name or relative path=w1756) -> (appended path=w1765:path)
        n792 = Open/Create/Replace File(file path (use dialog)=w1765, error in=w1759, operation (0:open)=T63."replace or create") -> (refnum out=w1762:refnum<file>, error out=w1758:errorcluster)  [unwired: 4 out]
        n793 = Write to Binary File(file (use dialog)=w1762, data=w1763, error in=w1758) -> (refnum out=w1760:refnum<file>, error out=w1761:errorcluster)  [unwired: 4 out]
        n794 = Close File(refnum=w1760, error in=w1761) -> (error out=w1757:errorcluster)  [unwired: 1 out]
      }
    }
    n795 = local read "App Running"() -> (w1754:bool)
    n796 = Wait Until Next ms Multiple(millisecond multiple=u32 2000) -> ()  [unwired: 1 out]
    n797 = call "Error Logger.vi"("error in (no error)"=w1748) -> ("error out"=w1747:errorcluster)  [unwired: 1 in, 9 out]
    n798 = Not(x=w1754) -> (.not. x?=w1745:bool)
  }
  n799 = Obtain Queue(element data type="", error in (no error)=w6) -> (queue out=w84:refnum<queue>, error out=w83:errorcluster)  [unwired: 2 in, 2 out]
  n800 = while {
    shift-right: [w1769] -> _
    shift-left: w84 -> [w1772]
    shift-right: [w1770] -> _
    shift-left: w83 -> [w1771]
    tunnel: [w1767] -> w82
    stop <- w1767 stop-if-true
    # "Archive Voltage Readings"
    n801 = Get Queue Status(queue=w1772, error in (no error)=w1771) -> (queue out=w1775:refnum<queue>, error out=w1776:errorcluster, # elements in queue=w1774:i32)  [unwired: 6 out]
    n802 = Wait Until Next ms Multiple(millisecond multiple=u32 2000) -> ()  [unwired: 1 out]
    n803 = Greater Than 0?(x=w1774) -> (x > 0?=w1773:bool)
    n804 = case shown="True" w1773 {
      tunnel: w1775 -> [w1780 w1789]
      tunnel: w1776 -> [w1779 w1788]
      tunnel: [w1779 w1786] -> w1777
      tunnel: [w1780 w1787] -> w1769
      frame #0 {
        n805 = Wait Until Next ms Multiple(millisecond multiple=u32 100) -> ()  [unwired: 1 out]
      }
      frame #1 {
        n806 = Flush Queue(queue=w1789, error in (no error)=w1788) -> (queue out=w1787:refnum<queue>, remaining elements=w1785:string[], error out=w1782:errorcluster)
        n807 = Concatenate Strings(w1785) -> (w1784:string)
        n808 = call "Save Text Data.vi"("error in"=w1782, "LogFile Type"=LogFileType."Volts", "String"=w1784) -> ("error out"=w1786:errorcluster)  [unwired: 1 in, 1 out]
      }
    }
    n809 = local read "App Running"() -> (w1778:bool)
    n810 = Not(x=w1778) -> (.not. x?=w1767:bool)
    n811 = call "Error Logger.vi"("error in (no error)"=w1777) -> ("error out"=w1770:errorcluster)  [unwired: 1 in, 9 out]
  }
  n812 = while {
    shift-right: [w1792] -> _
    shift-left: w84 -> [w1794]
    shift-right: [w1791] -> _
    shift-left: w83 -> [w1793]
    tunnel: [w1790] -> w81
    stop <- w1790 stop-if-true
    # "Collect Voltage Readings"
    n813 = call "App Status Globals.vi"("App Status Actions"=App_Status_Actions."Get Status") -> ("App Status Out"=w1798:T58)  [unwired: 5 in, 9 out]
    n814 = Unbundle By Name(w1798) -> ("Voltage Logging"=w1796:bool)
    n815 = local read "Volt Logger Time"() -> (w1795:u32)
    n816 = case shown="False" w1796 {
      tunnel: w1794 -> [w1801 w1806]
      tunnel: w1793 -> [w1800 w1805]
      tunnel: [w1801 w1803] -> w1792
      tunnel: [w1800 w1802] -> w1791
      frame #0 {
      }
      frame #1 {
        n817 = local read "L1 Cmd  Volts"() -> (w1810:dbl[])
        n818 = local read "L2 Cmd  Volts"() -> (w1809:dbl[])
        n819 = local read "DAQ Volts"() -> (w1808:dbl[])
        n820 = Build Array (concatenate)(w1810, w1809, w1808) -> (w1807:dbl[])
        n821 = call "Data 2 Record.vi"("Data"=w1807) -> ("Records"=w1804:string)  [unwired: 2 in, 8 out]
        n822 = Enqueue Element(queue=w1806, element=w1804, error in (no error)=w1805) -> (queue out=w1803:refnum<queue>, error out=w1802:errorcluster)  [unwired: 2 out]
      }
    }
    n823 = Wait Until Next ms Multiple(millisecond multiple=w1795) -> ()  [unwired: 1 out]
    n824 = local read "App Running"() -> (w1799:bool)
    n825 = Not(x=w1799) -> (.not. x?=w1790:bool)
  }
  n826 = Obtain Notifier(name (unnamed)="Command & Stiffness Changes", notification data type=w3, error in (no error)=w6) -> (notifier out=w2:refnum<notifier>, error out=w4:errorcluster)  [unwired: 1 in, 1 out]
  n827 = while {
    shift-right: [w1818] -> _
    shift-left: w5 -> [w1822]
    tunnel: w3 -> [w1816]
    shift-right: [w1814] -> _
    shift-left: w2 -> [w1815]
    shift-right: [w1812] -> _
    shift-left: w4 -> [w1821]
    tunnel: [w1811] -> w1
    stop <- w1811 stop-if-true
    n828 = Dequeue Element(queue=w1822, timeout in ms (-1)=2000, error in (no error)=w1821) -> (queue out=w1818:refnum<queue>, element=w1817:T29, timed out?=w1819:bool, error out=w1813:errorcluster)
    n829 = case shown="False" w1819 {
      tunnel: w1817 -> [w1824 _]
      tunnel: w1816 -> [w1829 _]
      tunnel: w1815 -> [w1828 w1855]
      tunnel: [w1827 w1855] -> w1814
      tunnel: w1813 -> [w1826 w1854]
      tunnel: [w1825 w1854] -> w1812
      frame #0 {
        n830 = case shown="\"Stiffness Update\"" w1824 {
          selector: w1824 -> [w1835 w1843 w1851]
          tunnel: w1829 -> [w1837 w1845 w1853]
          tunnel: w1828 -> [w1834 w1842 w1850]
          tunnel: [w1833 w1841 w1849] -> w1827
          tunnel: w1826 -> [w1832 w1840 w1848]
          tunnel: [w1831 w1839 w1847] -> w1825
          frame #0 {
            n831 = local read "Stiffness Jacobian Column"() -> (w1836:T3[])
            n832 = Bundle By Name(cluster=w1837, "Command || Stiffness Update"=w1835, "Stiffness"=w1836) -> (w1830:T28)
            n833 = Send Notification(notification=w1830, notifier=w1834, error in (no error)=w1832) -> (notifier out=w1833:refnum<notifier>, error out=w1831:errorcluster)
          }
          frame #1 {
            n834 = local read "Current Target"() -> (w1844:T5[])
            n835 = Bundle By Name(cluster=w1845, "Command || Stiffness Update"=w1843, "Target"=w1844) -> (w1838:T28)
            n836 = Send Notification(notification=w1838, notifier=w1842, error in (no error)=w1840) -> (notifier out=w1841:refnum<notifier>, error out=w1839:errorcluster)
          }
          frame #2 {
            n837 = local read "Iterative Target"() -> (w1852:T5[])
            n838 = Bundle By Name(cluster=w1853, "Command || Stiffness Update"=w1851, "Target"=w1852) -> (w1846:T28)
            n839 = Send Notification(notification=w1846, notifier=w1850, error in (no error)=w1848) -> (notifier out=w1849:refnum<notifier>, error out=w1847:errorcluster)
          }
        }
      }
      frame #1 {
      }
    }
    n840 = local read "App Running"() -> (w1823:bool)
    n841 = Not(x=w1823) -> (.not. x?=w1811:bool)
  }
  n842 = Compound Arithmetic op=AND(w94, w100, w99, w98, w97, w96, w95, w1, w82, w81) -> (w93:bool)
  n843 = flat-sequence {
    tunnel: w93 -> [w1858]
    frame #0 {
      n844 = local write "All Stopped"(w1858) -> ()
      n845 = call "NoArgumentsLauncher.vi"("Application"=NoPanelAppTypes."Control Loops", "Application Launcher Actions"=Launcher_Actions."Stop") -> ()  [unwired: 1 in, 9 out]
    }
  }
